vi "GUI_Scopes_v3.0.1.vi"() -> ()   [LabVIEW 2013]
uses:
  Device Drivers/PXIdigitizer/impedance_Enum_TypDEf.ctl
  Device Drivers/PXIdigitizer/coupling_Enum_TypDef.ctl
  Shared/type definition/trace_TypDef.ctl
  Device Drivers/shared/scopeTraceInfo_TypDEf.ctl
  Device Drivers/PXIdigitizer/mode_TypDef.ctl
  Device Drivers/PXIdigitizer/SignalFormat_TypDef.ctl
  Device Drivers/PXIdigitizer/triggerwindowmode2_TypDef.ctl
  Device Drivers/PXIdigitizer/TriggerSource_TypDef.ctl
  Shared/Device Driver/positive_negatice2_typDef.ctl
  Device Drivers/PXIdigitizer/coupling_TypDef.ctl
  Device Drivers/PXIdigitizer/TVEvent_TypDef.ctl
  Device Drivers/PXIdigitizer/Polarity_TypDEf.ctl
  Shared/Device Driver/OnOffTypeDef.ctl
  Device Drivers/PXIdigitizer/subVis/Trigger.DigitalSource_TypDEf.ctl
  Device Drivers/ScopeAnalysis/SubVis/method_TypDef.ctl
  Device Drivers/PXIdigitizer/subVis/channels_TypDef.ctl
  commandForScopeTrace.ctl
  <vilib>/Analysis/1siggen.llb/Ramp Pattern by Delta.vi
  <vilib>/Analysis/NI_AALBase.lvlib
panel:
  out "channelNames":refnum<vi>[](array[refnum])
  out "Number of channels":i32=8
  out "basic sub.":string="wait>>coupling.Channel1,coupling.Channel0,coupling.Channel2,coupling.Channel3,coupling.Channel4,coupling.Channel5,coupling.Channel6,coupling.Channel7,offset.Channel1,offset.Channel0,offset.Channel2,offset.Channel3,offset.Channel4,offset.Channel5,offset.Channel6,offset.Channel7,verticalrange.Channel1,verticalrange.Channel0,verticalrange.Channel2,verticalrange.Channel3,verticalrange.Channel4,verticalrange.Channel5,verticalrange.Channel6,verticalrange.Channel7,channelenabled.Channel1,channelenabled.Channel0,channelenabled.Channel2,channelenabled.Channel3,channelenabled.Channel4,channelenabled.Channel5,channelenabled.Channel6,channelenabled.Channel7,probeattenuation.Channel1,probeattenuation.Channel0,probeattenuation.Channel2,probeattenuation.Channel3,probeattenuation.Channel4,probeattenuation.Channel5,probeattenuation.Channel6,probeattenuation.Channel7,impedance.Channel1,impedance.Channel0,impedance.Channel2,impedance.Channel3,impedance.Channel4,impedance.Channel5,impedance.Channel6,impedance.Channel7,Names.Channel0,Names.Channel1,Names.Channel2,Names.Channel3,Names.Channel4,Names.Channel5,Names.Channel6,Names.Channel7,channelenabled.Channel0,channelenabled.Channel1,channelenabled.Channel2,channelenabled.Channel3,channelenabled.Channel4,channelenabled.Channel5,channelenabled.Channel6,channelenabled.Channel7,save,Horizontal.Enforce Realtime,Horizontal.Actual Record Length,Horizontal.Min Record Length,Horizontal.Actual Sample Rate,Horizontal.Min Sample Rate,Trigger.DC Restore,Trigger.Window Mode,Trigger.Polarity,Trigger.TV Event,Trigger.Coupling,Trigger.Slope,Trigger.AnalogSource,Trigger.High Level,Trigger.Low Level,Trigger.Hysteresis,Trigger.Delay,Trigger.Holdoff,Trigger.Signal Format,Trigger.Line Number,Trigger.Mode,Trigger.DigitalSource,"
  out "Channel NAmes":string[](array[string])
  out "show3 array":refnum<vi>[](array[refnum])
  out "showAll array":refnum<vi>[](array[refnum])
  out "enabled array":refnum<vi>[](array[refnum])
  out "wavegaph array":refnum<vi>[](array[refnum])
  out "traces array":refnum<vi>[](array[refnum])
  in  "save":T1
  out "horizontal ref":refnum<vi>[](array[refnum])
  out "Trigger ref":refnum<vi>[](array[refnum])
  out "indecator ref array":refnum<vi>[](array[refnum])
  in  "time to wait (TCP) 2":i32=10
  in  "plot":bool=TRUE
  out "ratio(h)":bool
  out "fixsize":bool
  in  "shotnumber":i32
  out "error (h)":bool
  in  "scopeTraceGUI.Channel7":T2
  in  "scopeTraceGUI.Channel6":T2
  in  "scopeTraceGUI.Channel4":T2
  in  "scopeTraceGUI.Channel3":T2
  in  "scopeTraceGUI.Channel5":T2
  in  "scopeTraceGUI.Channel2":T2
  out "Device Name (h)":string="TS-digitizer-1"
  in  "Main Tap":T4(tab)
  out "channel 1":waveform(dbl)(graph)
  in  "Tab Control":T5(tab)
  in  "coupling":T6=enum."DC"
  in  "channelenabled":enum16{"off", "on"}(ring)=enum."on"
  in  "offset":dbl
  in  "verticalrange":dbl=6.0
  in  "probeattenuation":dbl=1.0
  in  "impedance":T7=enum."50 ohms"
  in  "Channel":T8(ring)
  in  "ChannelRing":u16(ring) items=["Ch1", "Ch2", "Ch3", "Ch4", "Ch5", "Ch6", "Ch7", "Ch8"]
  in  "Horizontal.Min Sample Rate":dbl=6000000.0 step=1000000.0 format="%.2p"
  in  "Horizontal.Min Record Length":i32=10000 format="%.0p"
  out "Horizontal.Actual Record Length":i32=10000
  out "Horizontal.Actual Sample Rate":dbl=6000000.0 format="%.2p"
  in  "Horizontal.Enforce Realtime":T1=enum."on"
  out "time wimdow":dbl=0.0016666666666666668 format="%#_6p"
  out "resolution":dbl=1.6666666666666668e-07 format="%#_6p"
  in  "Trigger.Delay":dbl min=-0.001 max=0.001 step=1e-08 format="%#_12e"
  in  "Trigger.Coupling":T9=enum."DC" caption="Coupling"
  in  "Trigger.Mode":T10=enum."Digital Edge"
  in  "Trigger.Polarity":T11=enum."Positive" caption="Polarity"
  in  "Trigger.Line Number":i32=1
  in  "Trigger.Signal Format":T12 caption="Signal Format"
  in  "Trigger.DC Restore":T1
  in  "Trigger.TV Event":T13=enum."Any Line" caption="TV Event"
  in  "Trigger.Holdoff":dbl
  in  "Trigger.AnalogSource":T14
  in  "Trigger.Low Level":dbl=0.5
  in  "Trigger.Slope":T15 caption="Slope"
  in  "Trigger.High Level":dbl=1.0
  in  "Trigger.Hysteresis":dbl=0.05
  in  "Trigger.Window Mode":T16 caption="Window Mode"
  in  "Trigger.DigitalSource":T17=enum."PFI 1"
  out "Names.Channel2":string="Ch3"
  out "Names.Channel3":string="Ch4"
  out "Names.Channel4":string="Ch5"
  out "Names.Channel5":string="Ch6"
  out "Names.Channel6":string="Ch7"
  out "Names.Channel7":string="Ch8"
  in  "show.2":T8(ring)=enum."Channel1"
  in  "show.Channel0":bool=TRUE
  in  "show.Channel1":bool=TRUE
  in  "show.Channel2":bool
  in  "show.Channel3":bool
  in  "show.Channel4":bool
  in  "show.Channel5":bool
  in  "show.Channel6":bool
  in  "show.Channel7":bool
  in  "channelenabled.Channel0":bool=TRUE
  in  "Y scale from range":bool
  in  "channelenabled.Channel1":bool=TRUE
  in  "channelenabled.Channel2":bool=TRUE
  in  "channelenabled.Channel3":bool=TRUE
  in  "channelenabled.Channel4":bool=TRUE
  in  "channelenabled.Channel5":bool=TRUE
  in  "channelenabled.Channel6":bool=TRUE
  in  "channelenabled.Channel7":bool=TRUE
  in  "show.1":T8(ring)
  in  "Display":enum32{"All", "3Channels"}(radio)
  out "Names.Channel0":string="Ch1"
  out "Names.Channel1":string="Ch2"
  in  "Calculations.Additional.Analysis2":dbl=0.5
  in  "Calculations.Additional.Analysis1":dbl=0.5
  in  "Calculations.Method.Analysis2":T18 caption="Method"
  in  "Calculations.Linked.Analysis2":T19
  out "Measurements.Analysis2":dbl=0.5
  in  "Calculations.Method.Analysis1":T18 caption="Method"
  in  "Calculations.Linked.Analysis1":T19
  out "Measurements.Analysis1":dbl=0.5
  in  "scopeTraceGUI.Channel0":T2
  in  "scopeTraceGUI.Channel1":T2
  out "channel 0":waveform(dbl)(graph)
  out "All Channel":waveform(dbl)[](graph)
  out "local Port":u16=65442
  out "port or service name":u16=65445
  out "Remote Host":string="192.168.10.21"
  in  "timeout ms (slow resp)":i32=500
  in  "reset":bool
  out "image con closed":bool
  out "image \nconnection":bool
  out "image con closed 2":bool
  out "All Devices (h)":string[](array[string])=["PIXIFake", "TREX PXI fast", "TREX PXI slow", "TS-digitizer-1"]
  in  "time to wait (TCP)":i32=10
  out "error out":errorcluster
  out "connections (hidden)":variant[](array[variant])=[variant(refnum<k16> refnum), variant(refnum<k16> refnum)]
  in  "time to wait (main loop)":i32=200
  out "Data String":string="coupling.Channel1,DC\r\ncoupling.Channel0,DC\r\ncoupling.Channel2,DC\r\ncoupling.Channel3,DC\r\ncoupling.Channel4,DC\r\ncoupling.Channel5,DC\r\ncoupling.Channel6,DC\r\ncoupling.Channel7,DC\r\noffset.Channel1,0.000000000000\r\noffset.Channel0,0.000000000000\r\noffset.Channel2,0.000000000000\r\noffset.Channel3,0.000000000000\r\noffset.Channel4,0.000000000000\r\noffset.Channel5,0.000000000000\r\noffset.Channel6,0.000000000000\r\noffset.Channel7,0.000000000000\r\nverticalrange.Channel1,6.000000000000\r\nverticalrange.Channel0,6.000000000000\r\nverticalrange.Channel2,6.000000000000\r\nverticalrange.Channel3,6.000000000000\r\nverticalrange.Channel4,6.000000000000\r\nverticalrange.Channel5,6.000000000000\r\nverticalrange.Channel6,6.000000000000\r\nverticalrange.Channel7,6.000000000000\r\nchannelenabled.Channel1,on\r\nchannelenabled.Channel0,on\r\nchannelenabled.Channel2,on\r\nchannelenabled.Channel3,on\r\nchannelenabled.Channel4,on\r\nchannelenabled.Channel5,on\r\nchannelenabled.Channel6,on\r\nchannelenabled.Channel7,on\r\nprobeattenuation.Channel1,1.000000000000\r\nprobeattenuation.Channel0,1.000000000000\r\nprobeattenuation.Channel2,1.000000000000\r\nprobeattenuation.Channel3,1.000000000000\r\nprobeattenuation.Channel4,1.000000000000\r\nprobeattenuation.Channel5,1.000000000000\r\nprobeattenuation.Channel6,1.000000000000\r\nprobeattenuation.Channel7,1.000000000000\r\nimpedance.Channel1,50 ohms\r\nimpedance.Channel0,50 ohms\r\nimpedance.Channel2,50 ohms\r\nimpedance.Channel3,50 ohms\r\nimpedance.Channel4,50 ohms\r\nimpedance.Channel5,50 ohms\r\nimpedance.Channel6,50 ohms\r\nimpedance.Channel7,50 ohms\r\nNames.Channel0,Ch1\r\nNames.Channel1,Ch2\r\nNames.Channel2,Ch3\r\nNames.Channel3,Ch4\r\nNames.Channel4,Ch5\r\nNames.Channel5,Ch6\r\nNames.Channel6,Ch7\r\nNames.Channel7,Ch8\r\nchannelenabled.Channel0,on\r\nchannelenabled.Channel1,on\r\nchannelenabled.Channel2,on\r\nchannelenabled.Channel3,on\r\nchannelenabled.Channel4,on\r\nchannelenabled.Channel5,on\r\nchannelenabled.Channel6,on\r\nchannelenabled.Channel7,on\r\nsave,off\r\nHorizontal.Enforce Realtime,on\r\nHorizontal.Actual Record Length,10000.000000000000\r\nHorizontal.Min Record Length,10000.000000000000\r\nHorizontal.Actual Sample Rate,6000000.000000000000\r\nHorizontal.Min Sample Rate,6000000.000000000000\r\nTrigger.DC Restore,off\r\nTrigger.Window Mode,Entering\r\nTrigger.Polarity,Positive\r\nTrigger.TV Event,Any Line\r\nTrigger.Coupling,DC\r\nTrigger.Slope,Positive\r\nTrigger.AnalogSource,Channel 0\r\nTrigger.High Level,1.000000000000\r\nTrigger.Low Level,0.500000000000\r\nTrigger.Hysteresis,0.050000000000\r\nTrigger.Delay,0.000000000000\r\nTrigger.Holdoff,0.000000000000\r\nTrigger.Signal Format,M-NTSC\r\nTrigger.Line Number,1.000000000000\r\nTrigger.Mode,Digital Edge\r\nTrigger.DigitalSource,PFI 1\r\n"
  in  "Local Saving Path":path
  out "concatenated string":string="wait>>coupling.Channel1,coupling.Channel0,coupling.Channel2,coupling.Channel3,coupling.Channel4,coupling.Channel5,coupling.Channel6,coupling.Channel7,offset.Channel1,offset.Channel0,offset.Channel2,offset.Channel3,offset.Channel4,offset.Channel5,offset.Channel6,offset.Channel7,verticalrange.Channel1,verticalrange.Channel0,verticalrange.Channel2,verticalrange.Channel3,verticalrange.Channel4,verticalrange.Channel5,verticalrange.Channel6,verticalrange.Channel7,channelenabled.Channel1,channelenabled.Channel0,channelenabled.Channel2,channelenabled.Channel3,channelenabled.Channel4,channelenabled.Channel5,channelenabled.Channel6,channelenabled.Channel7,probeattenuation.Channel1,probeattenuation.Channel0,probeattenuation.Channel2,probeattenuation.Channel3,probeattenuation.Channel4,probeattenuation.Channel5,probeattenuation.Channel6,probeattenuation.Channel7,impedance.Channel1,impedance.Channel0,impedance.Channel2,impedance.Channel3,impedance.Channel4,impedance.Channel5,impedance.Channel6,impedance.Channel7,Names.Channel0,Names.Channel1,Names.Channel2,Names.Channel3,Names.Channel4,Names.Channel5,Names.Channel6,Names.Channel7,channelenabled.Channel0,channelenabled.Channel1,channelenabled.Channel2,channelenabled.Channel3,channelenabled.Channel4,channelenabled.Channel5,channelenabled.Channel6,channelenabled.Channel7,save,Horizontal.Enforce Realtime,Horizontal.Actual Record Length,Horizontal.Min Record Length,Horizontal.Actual Sample Rate,Horizontal.Min Sample Rate,Trigger.DC Restore,Trigger.Window Mode,Trigger.Polarity,Trigger.TV Event,Trigger.Coupling,Trigger.Slope,Trigger.AnalogSource,Trigger.High Level,Trigger.Low Level,Trigger.Hysteresis,Trigger.Delay,Trigger.Holdoff,Trigger.Signal Format,Trigger.Line Number,Trigger.Mode,Trigger.DigitalSource,"
  out "error message":string
  out "Data Connection out":bool=TRUE
  # "enabled"
  # "show"
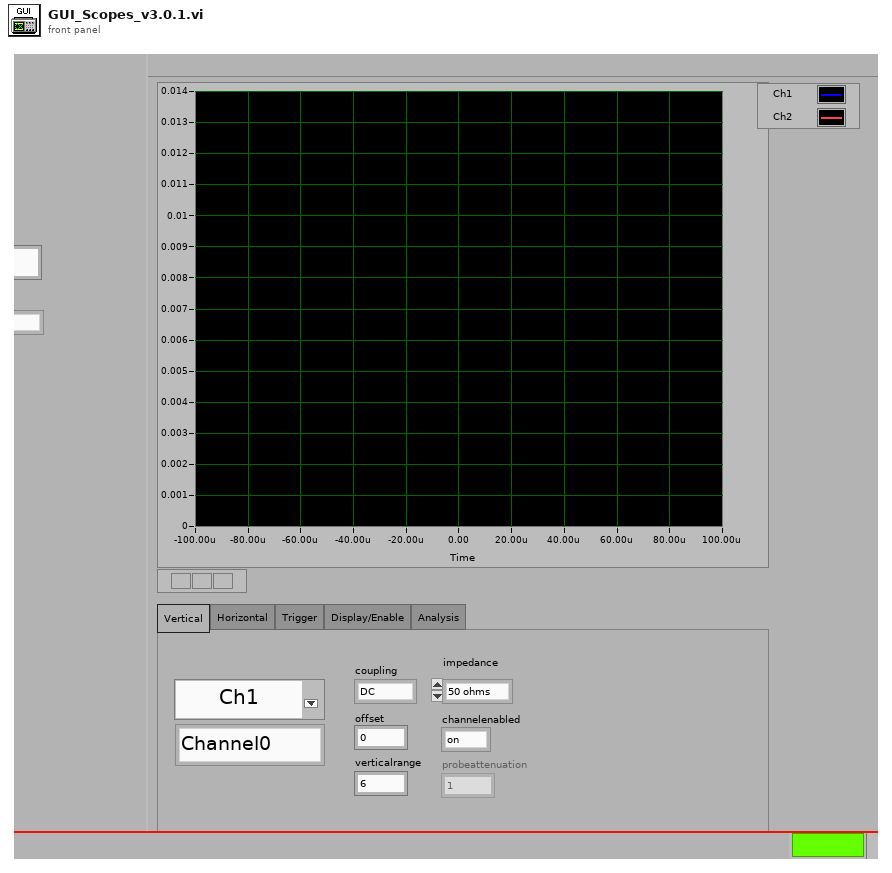
[diagram p1: front panel]
types:
  T1 = typedef "OnOffTypeDef.ctl" = enum16{"off", "on"}
  T2 = typedef "trace_TypDef.ctl" = cluster{"info":T3, "wfm":dbl[]}
  T3 = typedef "scopeTraceInfo_TypDEf.ctl" = cluster{"Name":string, "N":dbl, "t0":dbl, "dt":dbl, "offset":dbl, "gain":dbl, "coupling":string, "impedance":string, "range":dbl}
  T4 = enum32{"All Channels", "Network", "Internal", "Advanced"}
  T5 = enum32{"Vertical", "Horizontal", "Trigger", "Display/Enable", "Analysis"}
  T6 = typedef "coupling_Enum_TypDef.ctl" = enum16{"AC", "DC", "Ground"}
  T7 = typedef "impedance_Enum_TypDEf.ctl" = enum16{"1 mega ohm", "<NA>", "50 ohms"}
  T8 = enum16{"Channel0", "Channel1", "Channel2", "Channel3", "Channel4", "Channel5", "Channel6", "Channel7"}
  T9 = typedef "coupling_TypDef.ctl" = enum16{"AC", "DC", "HF Reject", "LF Reject", "AC Plus HF Reject"}
  T10 = typedef "mode_TypDef.ctl" = enum32{"Immediate", "Analog Edge", "Analog Window", "Analog Hysteresis", "Video", "Digital Edge"}
  T11 = typedef "Polarity_TypDEf.ctl" = enum16{"Negative", "Positive"}
  T12 = typedef "SignalFormat_TypDef.ctl" = enum16{"M-NTSC", "B/G-PAL", "SECAM", "M-PAL", "480i/59.94 fps", "480i/60 fps", "480p/59.94 Fps", "480p/60 Fps", "576i/50 fps", "576p/50 Fps", "720p/50 Fps", "720p/59.94 Fps", "720p/60 Fps", "1080i/50 fps", "1080i/59.94 fps", "1080i/60 fps", "1080p/24 Fps"}
  T13 = typedef "TVEvent_TypDef.ctl" = enum16{"Field 1", "Field 2", "Any Field", "Any Line", "Line Number"}
  T14 = typedef "TriggerSource_TypDef.ctl" = enum16{"Channel 0", "Channel 1", "Channel 2", "Channel 3", "Channel 4", "Channel 5", "Channel 6", "Channel 7", "External TRIG"}
  T15 = typedef "positive_negatice2_typDef.ctl" = enum16{"Positive", "Negative"}
  T16 = typedef "triggerwindowmode2_TypDef.ctl" = enum16{"Entering", "Leaving"}
  T17 = typedef "Trigger.DigitalSource_TypDEf.ctl" = enum16{"RTSI 0", "RTSI 1", "RTSI 2", "RTSI 3", "RTSI 4", "RTSI 5", "RTSI 6", "PFI 0", "PFI 1", "PFI 2", "PXI Star Trigger"}
  T18 = typedef "method_TypDef.ctl" = enum16{"n/a", "max", "min", "energy", "trigger", "maxtime", "mintime"}
  T19 = typedef "channels_TypDef.ctl" = enum16{"Channel0", "Channel1", "Channel2", "Channel3", "Channel4", "Channel5", "Channel6", "Channel7", "n/a"}
  T20 = typedef "commandForScopeTrace.ctl" = enum16{"get", "set", "init", "get ALL"}
  T21 = typedef "scopeTrace_TypDef.ctl" = cluster{"Info":cluster{"t0":dbl, "dt":dbl, "gain":dbl, "Name":string, "offset":dbl}, "Data":i16[]}
  T22 = cluster{"t0":dbl, "dt":dbl, "gain":dbl, "Name":string, "offset":dbl}
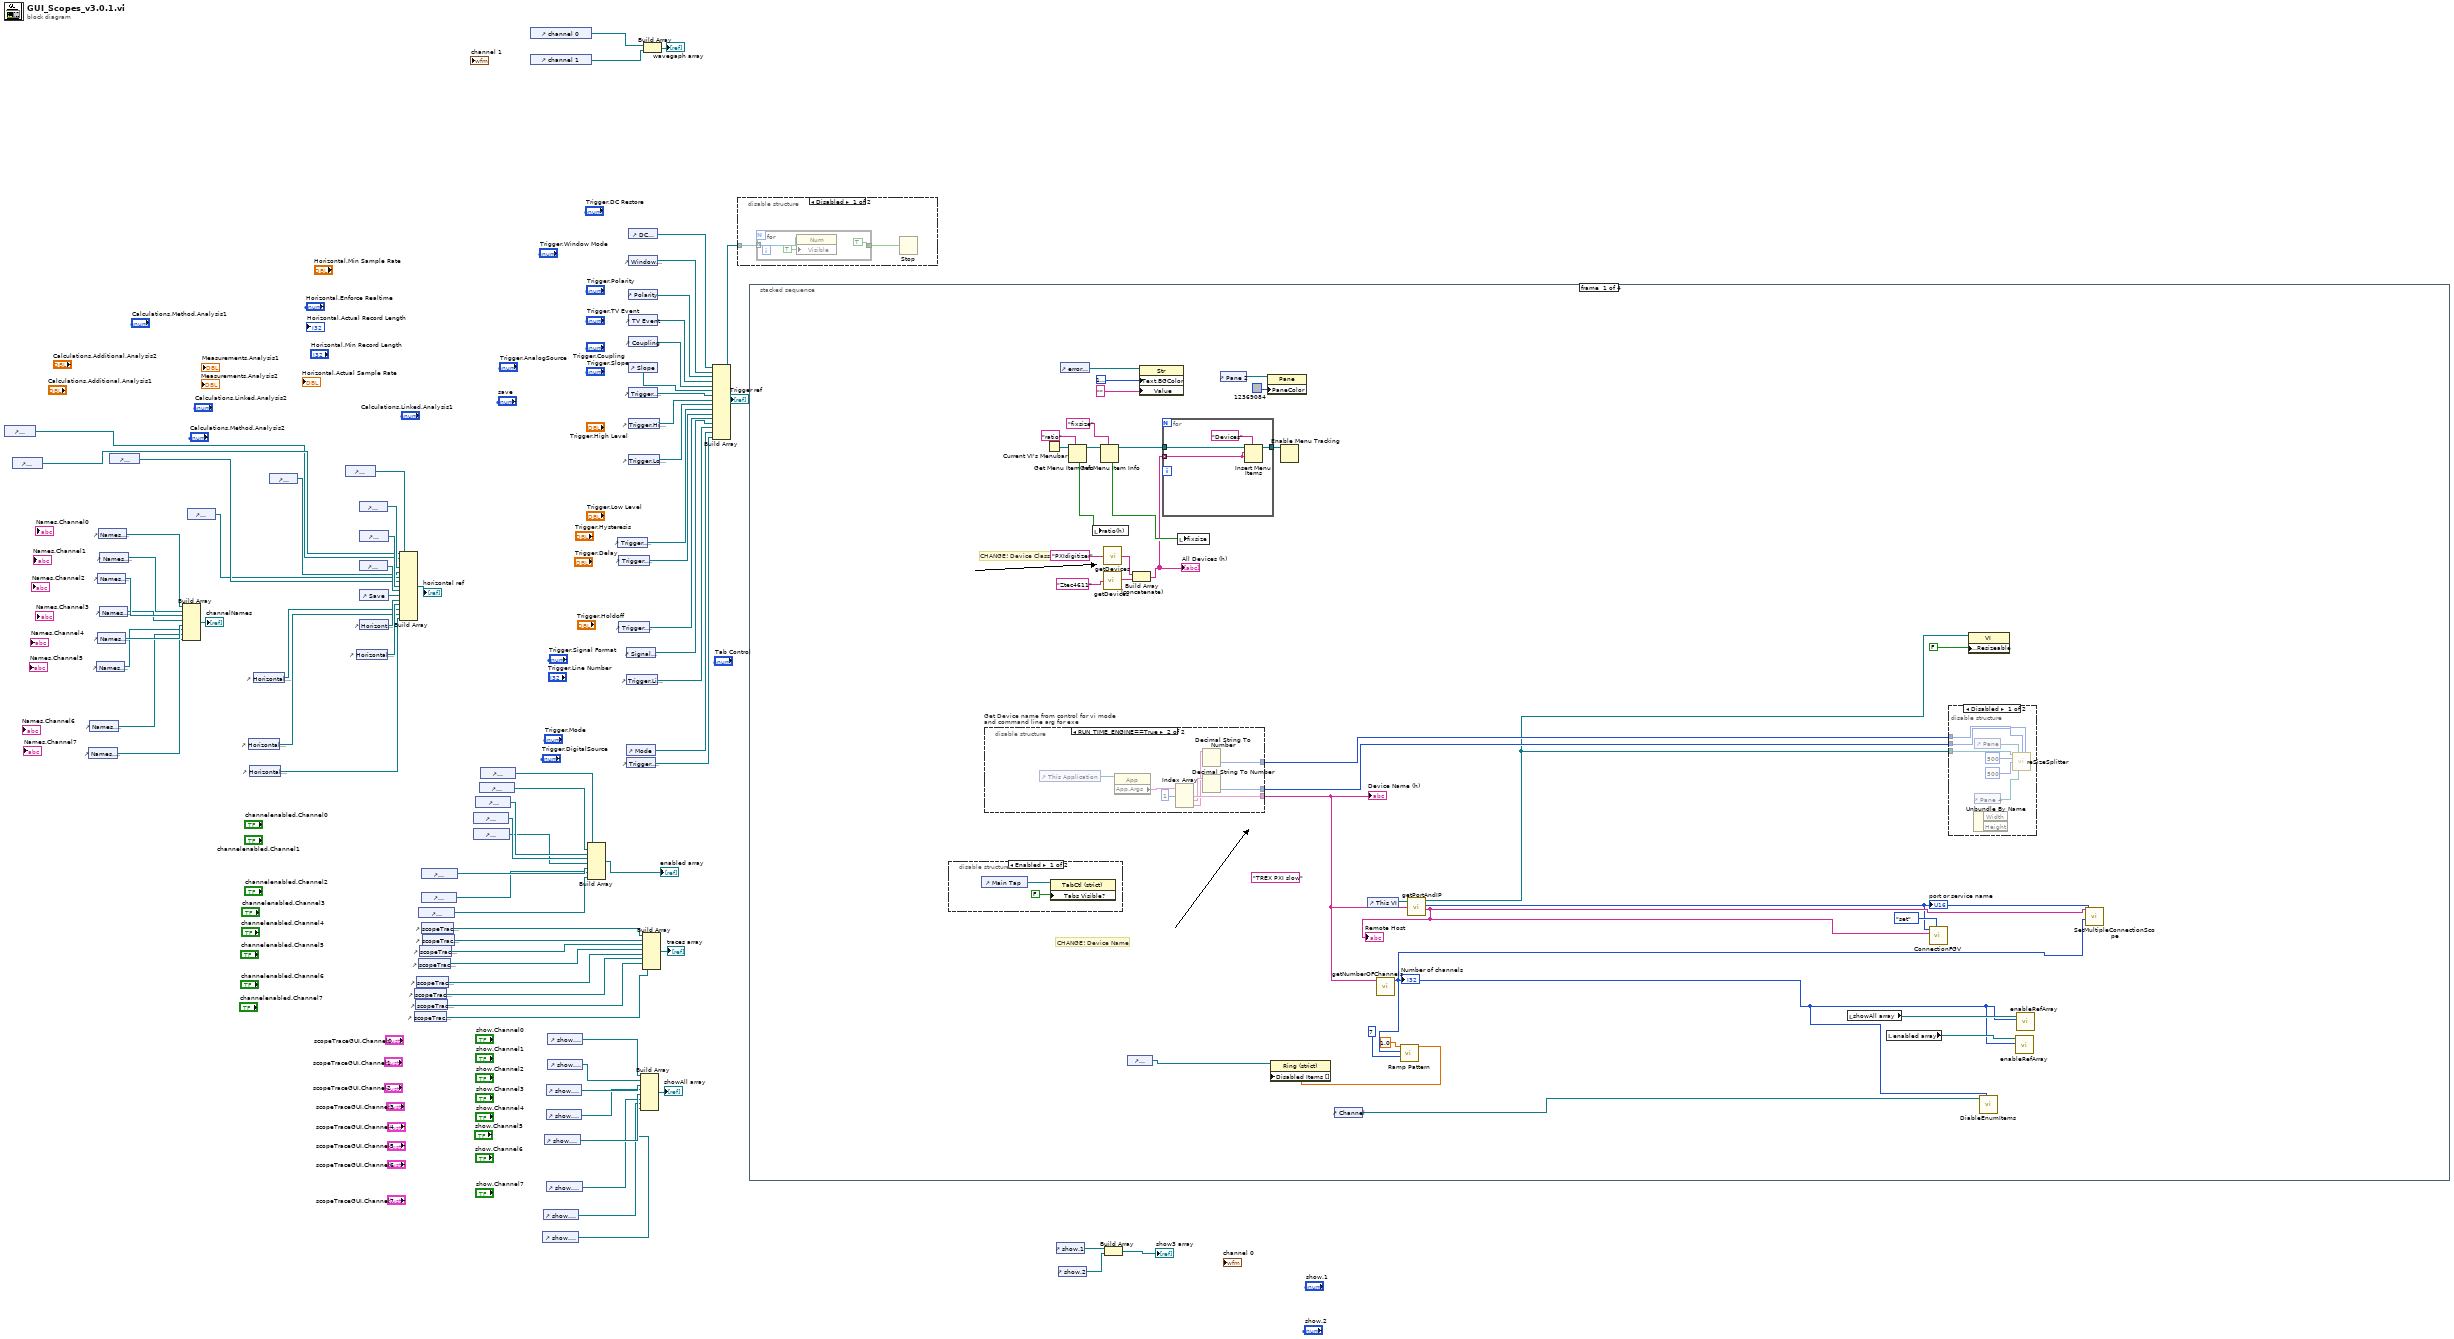
[diagram p0: block diagram]
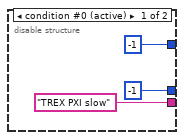
[diagram p5: hidden frame]
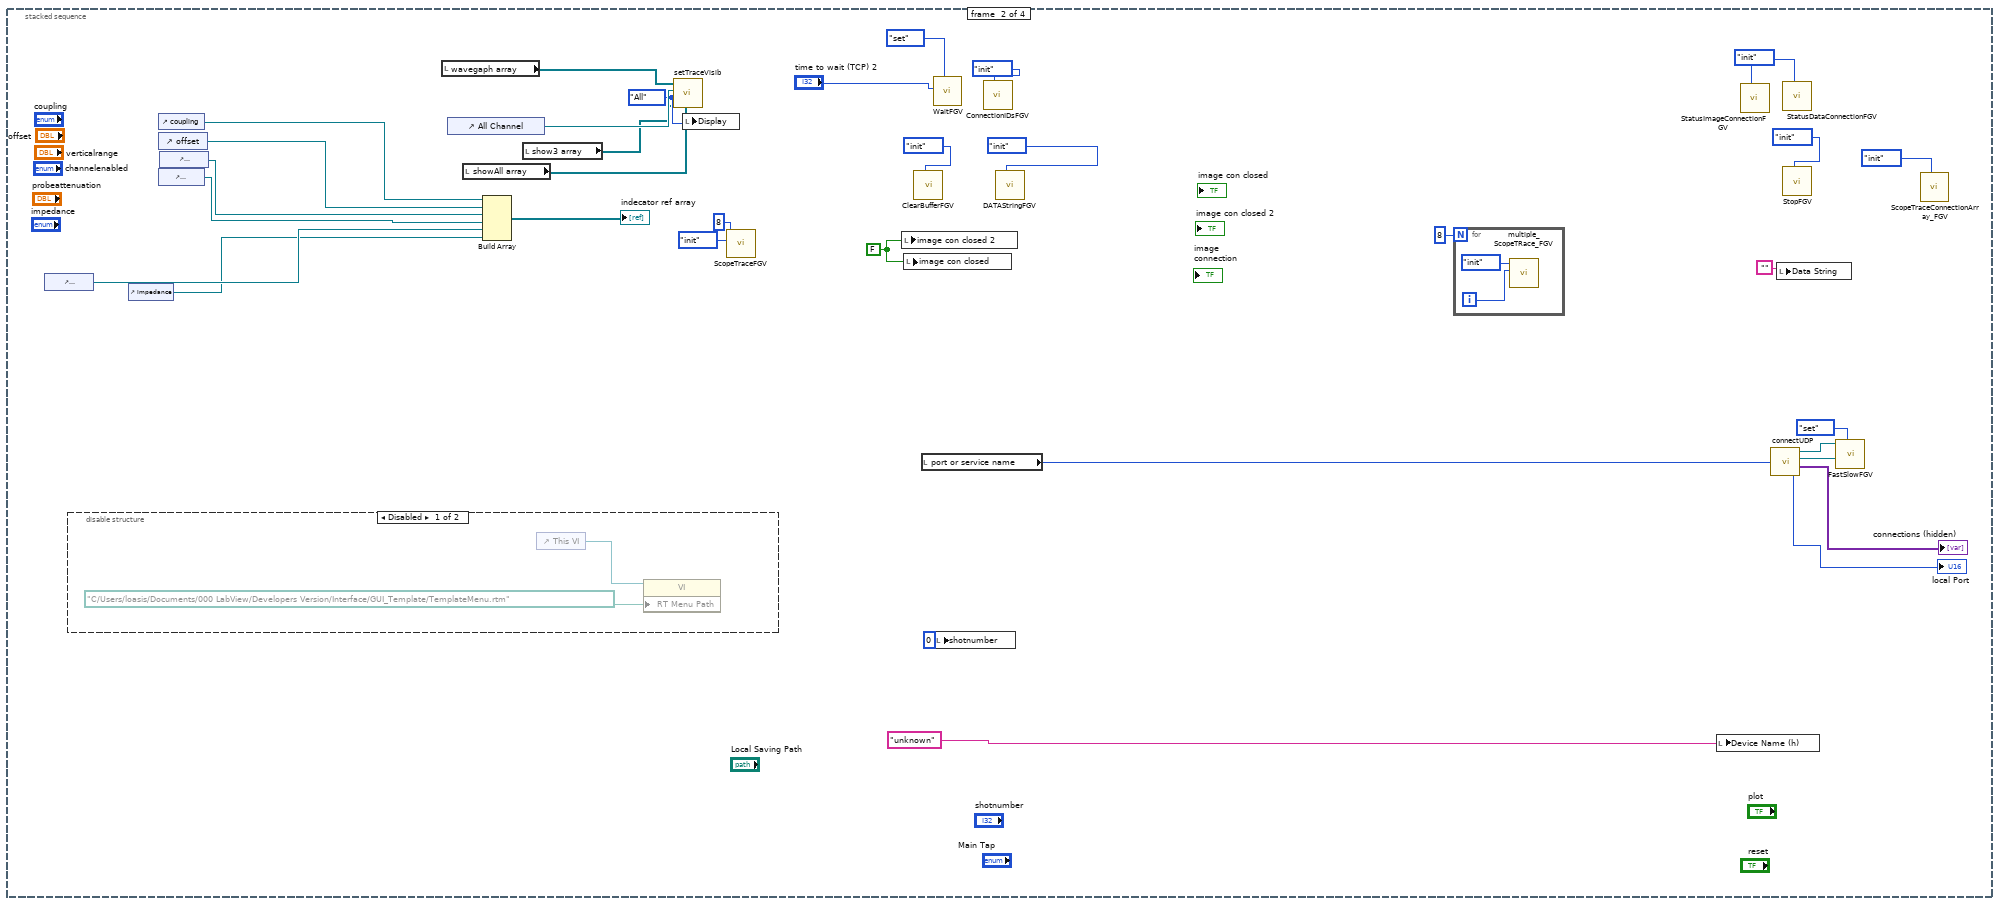
[diagram p6: hidden frame]
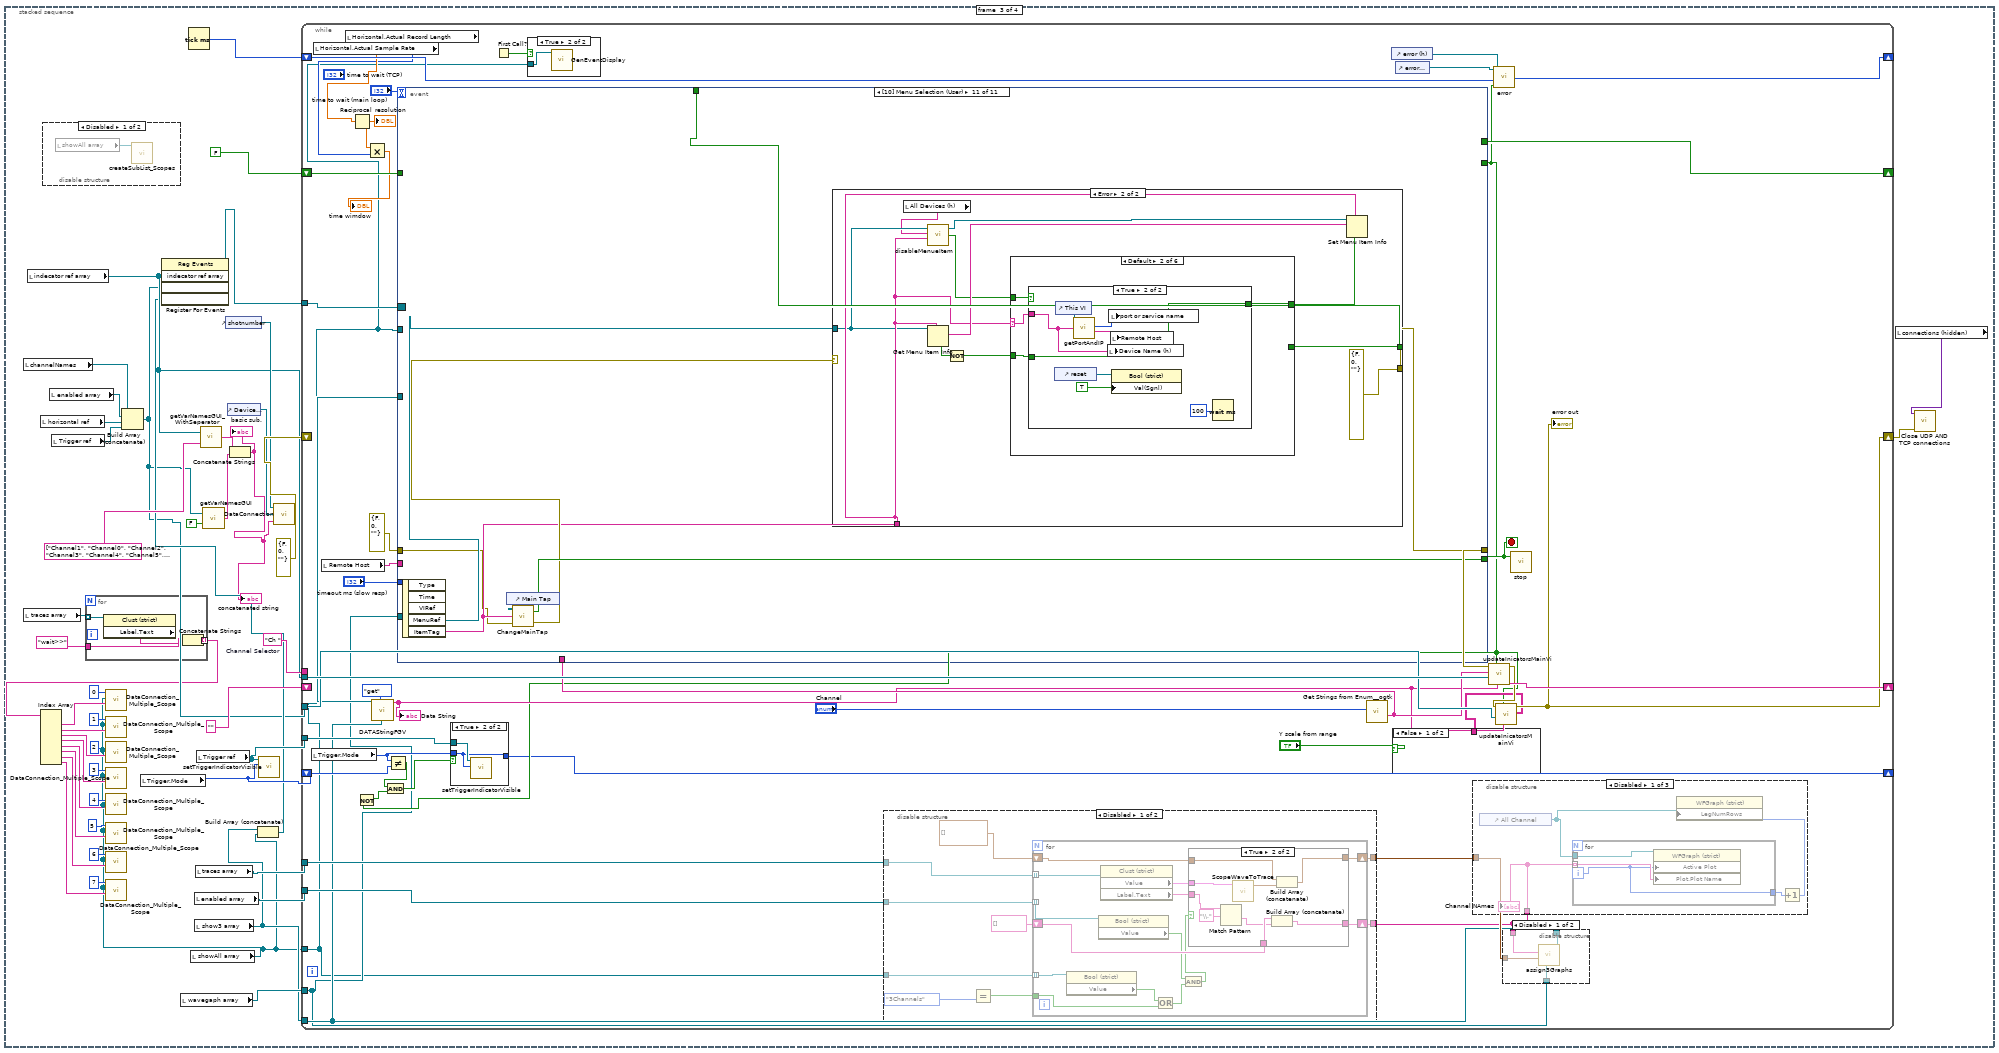
[diagram p8: hidden frame]
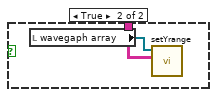
[diagram p17: hidden frame]
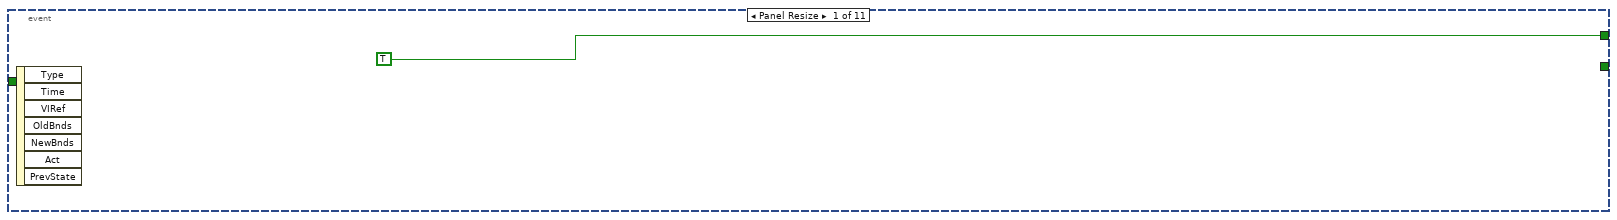
[diagram p18: hidden frame]
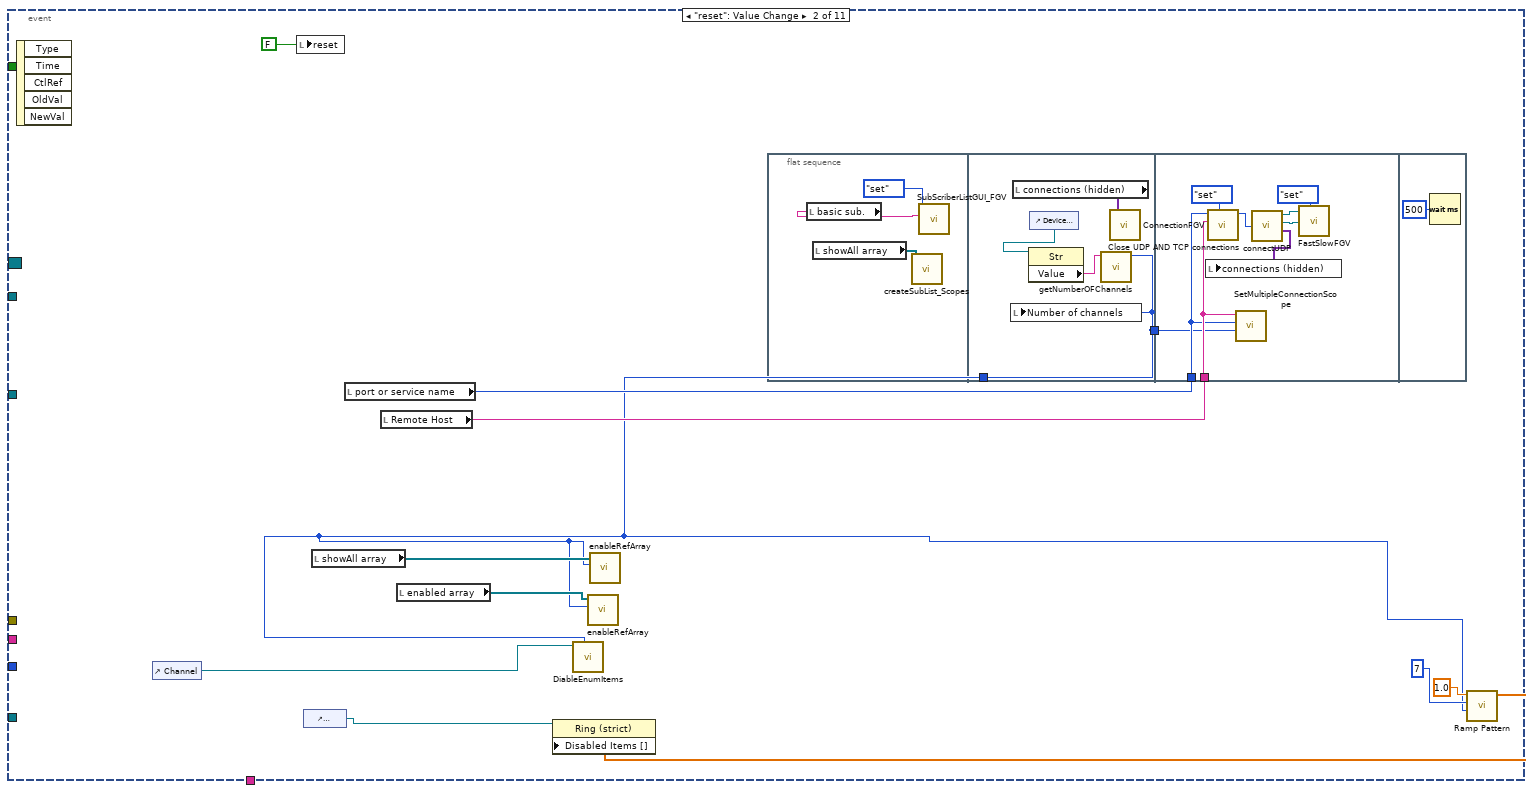
[diagram p19: hidden frame]
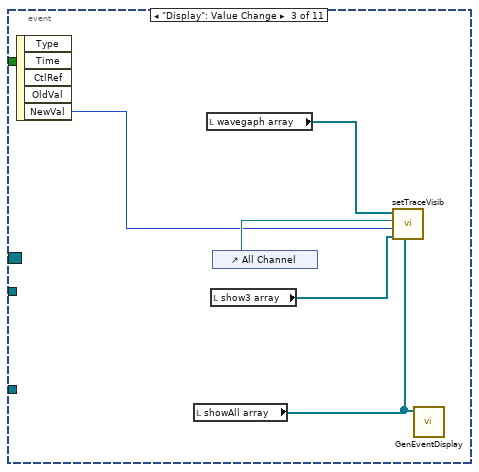
[diagram p20: hidden frame]
diagram:
  n1 = control-ref of="Calculations.Additional.Analysis1"() -> (w1:refnum<vi>)
  n2 = control-ref of="Calculations.Additional.Analysis2"() -> (w2:refnum<vi>)
  n3 = control-ref of="Names.Channel7"() -> (w11:refnum<vi>)
  n4 = control-ref of="Names.Channel6"() -> (w12:refnum<vi>)
  n5 = control-ref of="Names.Channel5"() -> (w13:refnum<vi>)
  n6 = control-ref of="Names.Channel2"() -> (w16:refnum<vi>)
  n7 = control-ref of="Names.Channel4"() -> (w14:refnum<vi>)
  n8 = control-ref of="Names.Channel0"() -> (w18:refnum<vi>)
  n9 = control-ref of="Names.Channel3"() -> (w15:refnum<vi>)
  n10 = control-ref of="Names.Channel1"() -> (w17:refnum<vi>)
  n11 = control-ref of="Measurements.Analysis1"() -> (w7:refnum<vi>)
  n12 = Build Array(w18, w17, w16, w15, w14, w13, w12, w11) -> (→"channelNames":refnum<vi>[])
  n13 = control-ref of="LinkedChannel.M2"() -> (w4:refnum<vi>)
  n14 = control-ref of="Horizontal.Actual Sample Rate"() -> (w56:refnum<vi>)
  n15 = control-ref of="Horizontal.Min Sample Rate"() -> (w54:refnum<vi>)
  n16 = control-ref of="Horizontal.Min Record Length"() -> (w57:refnum<vi>)
  n17 = control-ref of="LinkedChannel.M2"() -> (w5:refnum<vi>)
  n18 = control-ref of="Measurements.Analysis2"() -> (w3:refnum<vi>)
  n19 = control-ref of="Horizontal.Actual Record Length"() -> (w58:refnum<vi>)
  n20 = control-ref of="Calculations.Method.Analysis2"() -> (w6:refnum<vi>)
  n21 = control-ref of="Calculations.Method.Analysis1"() -> (w9:refnum<vi>)
  n22 = control-ref of="LinkedChannel.M1"() -> (w8:refnum<vi>)
  n23 = control-ref of="Save"() -> (w52:refnum<vi>)
  n24 = control-ref of="Horizontal.Enforce Realtime"() -> (w59:refnum<vi>)
  n25 = Build Array(w2, w1, w3, w6, w5, w4, w7, w8, w9, w52, w59, w58, w57, w56, w54) -> (→"horizontal ref":refnum<vi>[])
  n26 = control-ref of="scopeTrace.Channel7"() -> (w43:refnum<vi>)
  n27 = control-ref of="scopeTrace.Channel5"() -> (w45:refnum<vi>)
  n28 = control-ref of="scopeTrace.Channel6"() -> (w44:refnum<vi>)
  n29 = control-ref of="scopeTrace.Channel4"() -> (w46:refnum<vi>)
  n30 = control-ref of="scopeTrace.Channel3"() -> (w47:refnum<vi>)
  n31 = control-ref of="channelenabled.Channel7"() -> (w34:refnum<vi>)
  n32 = control-ref of="scopeTrace.Channel2"() -> (w48:refnum<vi>)
  n33 = control-ref of="channelenabled.Channel6"() -> (w35:refnum<vi>)
  n34 = control-ref of="channelenabled.Channel5"() -> (w36:refnum<vi>)
  n35 = control-ref of="scopeTrace.Channel0"() -> (w33:refnum<vi>)
  n36 = control-ref of="scopeTrace.Channel1"() -> (w32:refnum<vi>)
  n37 = control-ref of="channelenabled.Channel3"() -> (w38:refnum<vi>)
  n38 = control-ref of="channelenabled.Channel4"() -> (w37:refnum<vi>)
  n39 = control-ref of="channelenabled.Channel2"() -> (w39:refnum<vi>)
  n40 = control-ref of="channelenabled.Channel1"() -> (w40:refnum<vi>)
  n41 = control-ref of="channelenabled.Channel0"() -> (w42:refnum<vi>)
  n42 = control-ref of="channel 1"() -> (w19:refnum<vi>)
  n43 = control-ref of="channel 0"() -> (w50:refnum<vi>)
  n44 = control-ref of="show.Channel7"() -> (w24:refnum<vi>)
  n45 = control-ref of="show.Channel6"() -> (w25:refnum<vi>)
  n46 = control-ref of="show.Channel4"() -> (w27:refnum<vi>)
  n47 = control-ref of="show.Channel2"() -> (w29:refnum<vi>)
  n48 = control-ref of="show.Channel3"() -> (w28:refnum<vi>)
  n49 = control-ref of="show.Channel5"() -> (w26:refnum<vi>)
  n50 = control-ref of="show.Channel0"() -> (w31:refnum<vi>)
  n51 = control-ref of="show.Channel1"() -> (w30:refnum<vi>)
  n52 = Build Array(w42, w40, w39, w38, w37, w36, w35, w34) -> (→"enabled array":refnum<vi>[])
  n53 = control-ref of="Trigger.Hysteresis"() -> (w66:refnum<vi>)
  n54 = control-ref of="Trigger.Holdoff"() -> (w64:refnum<vi>)
  n55 = control-ref of="Trigger.Delay"() -> (w65:refnum<vi>)
  n56 = control-ref of="Signal Format"() -> (w63:refnum<vi>)
  n57 = control-ref of="Trigger.Line Number"() -> (w62:refnum<vi>)
  n58 = control-ref of="Mode"() -> (w61:refnum<vi>)
  n59 = control-ref of="Trigger.DigitalSource"() -> (w60:refnum<vi>)
  n60 = control-ref of="DC Restore"() -> (w75:refnum<vi>)
  n61 = control-ref of="Window Mode"() -> (w74:refnum<vi>)
  n62 = control-ref of="Polarity"() -> (w73:refnum<vi>)
  n63 = control-ref of="TV Event"() -> (w72:refnum<vi>)
  n64 = control-ref of="Coupling"() -> (w71:refnum<vi>)
  n65 = control-ref of="Slope"() -> (w70:refnum<vi>)
  n66 = control-ref of="Trigger.AnalogSource"() -> (w69:refnum<vi>)
  n67 = control-ref of="Trigger.High Level"() -> (w68:refnum<vi>)
  n68 = control-ref of="Trigger.Low Level"() -> (w67:refnum<vi>)
  n69 = Build Array(w31, w30, w29, w28, w27, w26, w25, w24) -> (→"showAll array":refnum<vi>[])
  n70 = Build Array(w33, w32, w48, w47, w46, w45, w44, w43) -> (→"traces array":refnum<vi>[])
  n71 = Build Array(w50, w19) -> (→"wavegaph array":refnum<vi>[])
  n72 = Build Array(w75, w74, w73, w72, w71, w70, w69, w68, w67, w66, w65, w64, w63, w62, w61, w60) -> (w53:refnum<vi>[])
  "Trigger ref" <- w53
  n73 = disable-structure shown="Disabled" {
    disable-tunnel: w53 -> [w77 _]
    frame Disabled {
      n74 = for {
        tunnel: w77 -> [w80] mode=indexing
        tunnel: [TRUE] -> w76
        n75 = property class="Num"(reference=w80, "Visible"=TRUE) -> ()  [unwired: 1 in, 2 out]
      }
      n76 = Stop(stop? (T)=w76) -> ()
    }
    frame Enabled {
    }
  }
  n77 = stacked-sequence {
    frame #0 {
      (unwired) "TREX PXI slow" ("Device Name for vi mode")
      # "CHANGE! Device Name"
      # "CHANGE! Device Class"
      n78 = disable-structure shown="Enabled" {
        frame Enabled {
          n79 = control-ref of="Main Tap"() -> (w117:refnum<vi>)
          n80 = property class="TabCtl (strict)"(reference=w117, "Tabs Visible?"=FALSE) -> ()  [unwired: 1 in, 2 out]
        }
        frame Disabled {
        }
      }
      n81 = disable-structure "Get Device name from control for vi mode\nand command line arg for exe" shown="RUN_TIME_ENGINE==True" {
        disable-tunnel: ["TREX PXI slow" ("Device Name for vi mode") w136] -> w93
        disable-tunnel: [i16 -1 ("left") w133] -> w115
        disable-tunnel: [i16 -1 ("left") w132] -> w114
        frame condition #0 (active) {
        }
        frame condition #1 {
          n82 = control-ref of="This Application"() -> (w139:refnum<vi>)
          n83 = property class="App"(reference=w139) -> ("App.Args"=w138:string[])  [unwired: 1 in, 2 out]
          n84 = Index Array(array=w138, index #1=1 ("index")) -> (element #1=w136:string, element #2=w135:string, element #3=w134:string)  [unwired: 2 in]
          n85 = Decimal String To Number(string=w134) -> (number=w132:i32)  [unwired: 2 in, 1 out]
          n86 = Decimal String To Number(string=w135) -> (number=w133:i32)  [unwired: 2 in, 1 out]
        }
      }
      "Device Name (h)" <- w93
      n87 = Current VI's Menubar() -> (w108:refnum<k9>)
      n88 = control-ref of="error message"() -> (w102:refnum<vi>)
      n89 = Get Menu Item Info(7:"ratio" ("item tag"), 11:w108) -> (3:w106:refnum<k9>, 4:w107:bool)  [unwired: 1 in, 5 out]
      n90 = local write "ratio(h)"(w107) -> ()
      n91 = Get Menu Item Info(7:"fixsize" ("item tag"), 11:w106) -> (3:w98:refnum<k9>, 4:w104:bool)  [unwired: 1 in, 5 out]
      n92 = call "getDevices.vi"("Device Class"="Ztec4611") -> ("All Devices"=w82:string[])
      n93 = call "getDevices.vi"("Device Class"="PXIdigitizer") -> ("All Devices"=w83:string[])
      n94 = control-ref of="ChannelRing"() -> (w89:refnum<vi>)
      n95 = Build Array (concatenate)(w83, w82) -> (w81:string[])
      "All Devices (h)" <- w81
      n96 = property class="Str"(reference=w102, "Text.BGColor"=u32 16777238, "Value"="") -> ()  [unwired: 1 in, 2 out]
      n97 = for {
        tunnel: w98 -> [w121]
        tunnel: [w120] -> w97
        tunnel: w81 -> [w118] mode=indexing
        n98 = Insert Menu Items(5:"Devices" ("menu tag"), 7:w118, 8:w118, 9:w121) -> (3:w120:refnum<k9>)  [unwired: 2 in, 2 out]
      }
      n99 = local write "fixsize"(w104) -> ()
      n100 = control-ref of="Pane 2"() -> (w100:refnum<vi>)
      n101 = property class="Pane"(reference=w100, "PaneColor"=u32 12369084) -> ()  [unwired: 1 in, 2 out]
      n102 = Enable Menu Tracking(4:w97) -> ()  [unwired: 2 in, 2 out]
      n103 = control-ref of="Channel"() -> (w86:refnum<vi>)
      n104 = control-ref of="This VI"() -> (w113:refnum<vi>)
      n105 = call "getNumberOFChannels.vi"("Device Name for vi mode"=w93) -> ("Number of channels"=w85:i32)  [unwired: 10 in]
      "Number of channels" <- w85
      n106 = call-poly <vilib>:"Ramp Pattern.vi"("start"=7 ("x"), "end"=w85, "delta"=1.0) -> ("Ramp Pattern"=w87:dbl[])  [unwired: 6 in, 2 out]
      n107 = property class="Ring (strict)"(reference=w89, "Disabled Items []"=w87) -> ()  [unwired: 1 in, 2 out]
      n108 = call "getPortAndIP.vi"("Device Name"=w93, "This Vi"=w113) -> ("Remote Host"=w95:string, "port or service name"=w94:u16, "reference out"=w111:refnum<vi>)  [unwired: 2 in, 2 out]
      "port or service name" <- w94
      "Remote Host" <- w95
      n109 = local read "showAll array"() -> (w92:refnum<vi>[])
      n110 = local read "enabled array"() -> (w91:refnum<vi>[])
      n111 = call "ConnectionFGV.vi"("command"=enum16{"get", "set", "init"}."set", "Remote Host in"=w95, "port or service name in"=w94) -> ()  [unwired: 7 in, 2 out]
      n112 = disable-structure shown="Disabled" {
        disable-tunnel: w115 -> [w127 _]
        disable-tunnel: w114 -> [w126 _]
        disable-tunnel: w111 -> [w124 _]
        frame Disabled {
          n113 = Unbundle By Name() -> ()  [unwired: 1 in, 2 out]
          n114 = control-ref of="Pane"() -> (w128:refnum<vi>)
          n115 = control-ref of="Pane 4"() -> (w125:refnum<vi>)
          n116 = call "reSizeSplitter.vi"("this vi"=w124, "pane"=w128, "left"=w127, "top"=w126, "Width"=u32 500, "Height"=u32 500, "pane2"=w125) -> ()  [unwired: 8 in, 1 out]
        }
        frame Enabled {
        }
      }
      n117 = property class="VI"(reference=w111, "Front Panel.Resizeable"=FALSE ("Front Panel Window:Resizable")) -> ()  [unwired: 1 in, 2 out]
      n118 = call "DiableEnumItems.vi"("Number Of Channels"=w85, "Enum in"=w86) -> ()  [unwired: 10 in]
      n119 = call "enableRefArray.vi"("Number of channels"=w85, "showAll array"=w91) -> ()  [unwired: 10 in]
      n120 = call "enableRefArray.vi"("Number of channels"=w85, "showAll array"=w92) -> ()  [unwired: 10 in]
      n121 = call "SetMultipleConnectionScope.vi"("Number of Connections size"=w85, "port or service name"=w94, "Remote Host"=w95) -> ()  [unwired: 9 in]
    }
    frame #1 {
      w146 = enum32{"All", "3Channels"}."All" ("NewVal")
      w164 = enum16{"get", "set", "init"}."init" ("Command")
      w170 = FALSE ("new Device Data")
      n122 = control-ref of="probeattenuation"() -> (w155:refnum<vi>)
      n123 = disable-structure shown="Disabled" {
        frame Disabled {
          n124 = control-ref of="This VI"() -> (w176:refnum<vi>)
          n125 = property class="VI"(reference=w176, "RT Menu Path"=path "C:/Users/loasis/Documents/000 LabView/Developers Version/Interface/GUI_Template/TemplateMenu.rtm" ("Run-Time Menu Path")) -> ()  [unwired: 1 in, 2 out]
        }
        frame Enabled {
        }
      }
      n126 = control-ref of="Impedance"() -> (w149:refnum<vi>)
      n127 = control-ref of="coupling"() -> (w152:refnum<vi>)
      n128 = control-ref of="offset"() -> (w151:refnum<vi>)
      n129 = control-ref of="channelenabled"() -> (w154:refnum<vi>)
      n130 = control-ref of="verticalrange"() -> (w153:refnum<vi>)
      n131 = local read "wavegaph array"() -> (w148:refnum<vi>[])
      n132 = control-ref of="All Channel"() -> (w147:refnum<vi>)
      n133 = local read "showAll array"() -> (w144:refnum<vi>[])
      n134 = Build Array(w152, w151, w153, w154, w155, w149) -> (→"indecator ref array":refnum<vi>[])
      n135 = local read "show3 array"() -> (w145:refnum<vi>[])
      n136 = call "setTraceVisib.vi"("showAll array 2"=w144, "show3 array 3"=w145, "NewVal"=w146, "All Channel"=w147, "wavegaph array 2"=w148) -> ()  [unwired: 7 in]
      n137 = local write "Display"(w146) -> ()
      n138 = call "ScopeTraceFGV.vi"("command"=enum16{"get", "set", "init"}."init", "Nr."=8) -> ()  [unwired: 8 in, 2 out]
      n139 = local write "image con closed 2"(w170) -> ()
      n140 = local write "image con closed"(w170) -> ()
      n141 = call "ClearBufferFGV.vi"("Command"=enum16{"set", "get", "init"}."init") -> ()  [unwired: 10 in, 1 out]
      n142 = local read "port or service name"() -> (w160:u16)
      n143 = call "WaitFGV.vi"("Command"=enum16{"get", "set", "init"}."set", "milliseconds to wait"="time to wait (TCP) 2") -> ()  [unwired: 9 in, 1 out]
      n144 = local write "shotnumber"(0 ("shotnumber")) -> ()
      n145 = call "ConnectionIDsFGV.vi"("Command"=enum16{"add", "get", "init"}."init") -> ()  [unwired: 10 in, 1 out]
      n146 = call "DATAStringFGV.vi"("Command"=enum16{"get", "set", "init"}."init") -> ()  [unwired: 9 in, 2 out]
      n147 = for {
        N: 8 -> [_]
        i -> [w173]
        n148 = call "multiple_ScopeTRace_FGV.vi"("Nr."=w173, "command"=commandForScopeTrace."init") -> ()  [unwired: 9 in, 1 out]
      }
      n149 = local write "Device Name (h)"("unknown" ("Device Name")) -> ()
      n150 = call "StatusImageConnectionFGV.vi"("Command"=w164) -> ()  [unwired: 10 in, 1 out]
      n151 = call "connectUDP.vi"("port or service name NOT USED"=w160) -> ("fast ID (h)"=w159:refnum<k16>, "slow ID (h)"=w158:refnum<k16>, "connections (hidden)"=→"connections (hidden)":variant[], "local Port"=→"local Port":u16)
      n152 = local write "Data String"("") -> ()
      n153 = call "StatusDataConnectionFGV.vi"("Command"=w164) -> ()  [unwired: 10 in, 1 out]
      n154 = call "StopFGV.vi"("Command"=enum16{"set", "get", "init"}."init") -> ()  [unwired: 9 in, 2 out]
      n155 = call "FastSlowFGV.vi"("Command"=enum16{"get", "set", "init"}."set", "slow ID"=w158, "fast ID"=w159) -> ()  [unwired: 7 in, 2 out]
      n156 = call "ScopeTraceConnectionArray_FGV.vi"("Command"=enum16{"add", "get", "init"}."init") -> ()  [unwired: 9 in, 2 out]
    }
    frame #2 {
      w215 = "Ch "  # Channel Selector
      n157 = local read "channelNames"() -> (w177:refnum<vi>[])
      n158 = local read "traces array"() -> (w197:refnum<vi>[])
      n159 = local read "indecator ref array"() -> (w211:refnum<vi>[])
      n160 = local read "horizontal ref"() -> (w210:refnum<vi>[])
      n161 = disable-structure shown="Disabled" {
        frame Disabled {
          n162 = local read "showAll array"() -> (w225:refnum<vi>[])
          n163 = call "createSubList_Scopes.vi"("showAll array"=w225) -> ()  [unwired: 10 in, 1 out]
        }
        frame Enabled {
        }
      }
      n164 = local read "enabled array"() -> (w200:refnum<vi>[])
      n165 = local read "Trigger ref"() -> (w209:refnum<vi>[])
      n166 = for {
        tunnel: w197 -> [w229] mode=indexing
        tunnel: "wait>>" -> [w228]
        tunnel: [w226] -> w195 mode=indexing
        n167 = property class="Clust (strict)"(reference=w229) -> ("Label.Text"=w227:string)  [unwired: 1 in, 2 out]
        n168 = Concatenate Strings(w228, w227) -> (w226:string)
      }
      n169 = Index Array(array=w195) -> (element #1=w194:string, element #2=w193:string, element #3=w192:string, element #4=w191:string, element #5=w190:string, element #6=w179:string, element #7=w189:string, element #8=w188:string)  [unwired: 8 in]
      n170 = Build Array (concatenate)(w177, w200, w210, w209) -> (w198:refnum<vi>[])
      n171 = local read "Trigger.Mode"() -> (w207:T10)
      n172 = local read "wavegaph array"() -> (w203:refnum<vi>[])
      n173 = Tick Count (ms)() -> (millisecond timer value=w220:u32)
      n174 = local read "showAll array"() -> (w178:refnum<vi>[])
      n175 = call "DataConnection_Multiple_Scope.vi"("Image Subscriber list"=w194, "showAll array"=w178, "Nr."=0) -> ()  [unwired: 9 in]
      n176 = call "DataConnection_Multiple_Scope.vi"("Image Subscriber list"=w193, "showAll array"=w178, "Nr."=1) -> ()  [unwired: 9 in]
      n177 = call "DataConnection_Multiple_Scope.vi"("Image Subscriber list"=w192, "showAll array"=w178, "Nr."=2) -> ()  [unwired: 9 in]
      n178 = call "DataConnection_Multiple_Scope.vi"("Image Subscriber list"=w191, "showAll array"=w178, "Nr."=3) -> ()  [unwired: 9 in]
      n179 = call "DataConnection_Multiple_Scope.vi"("Image Subscriber list"=w190, "showAll array"=w178, "Nr."=4) -> ()  [unwired: 9 in]
      n180 = call "DataConnection_Multiple_Scope.vi"("Image Subscriber list"=w179, "showAll array"=w178, "Nr."=5) -> ()  [unwired: 9 in]
      n181 = call "DataConnection_Multiple_Scope.vi"("Image Subscriber list"=w189, "showAll array"=w178, "Nr."=6) -> ()  [unwired: 9 in]
      n182 = call "DataConnection_Multiple_Scope.vi"("Image Subscriber list"=w188, "showAll array"=w178, "Nr."=7) -> ()  [unwired: 9 in]
      n183 = local read "enabled array"() -> (w204:refnum<vi>[])
      n184 = local read "show3 array"() -> (w202:refnum<vi>[])
      n185 = local read "traces array"() -> (w205:refnum<vi>[])
      n186 = local read "Trigger ref"() -> (w206:refnum<vi>[])
      n187 = call "getVarNamesGUI_WithSeperator.vi"("Channels"=string[] ["Channel1", "Channel0", "Channel2", "Channel3", "Channel4", "Channel5", "Channel6", "Channel7"], "Array"=w211) -> ("String"=w213:string)
      n188 = call "getVarNamesGUI.vi"("start"=FALSE, "Array"=w198) -> ("String"=w212:string)
      n189 = control-ref of="shotnumber"() -> (w218:refnum<vi>)
      n190 = control-ref of="Device Name (h)"() -> (w217:refnum<vi>)
      n191 = Concatenate Strings(w213, w212) -> (w199:string)
      "concatenated string" <- w199
      "basic sub." <- w199
      n192 = Build Array (concatenate)(w202, w178) -> (w201:refnum<vi>[])
      n193 = register-events(w211, w198, w201) -> (reference out=w216:refnum<event-registration>)  [unwired: 2 in, 1 out]
      n194 = call "setTriggerIndicatorVisible.vi"("NewVal"=w207, "Trigger ref"=w206) -> ()  [unwired: 10 in]
      n195 = call "DataConnection.vi"("Subscriber list"=w199, "Device Name (h)"=w217, "shotnumber"=w218) -> ()
      n196 = while {
        shift-right: [w255] -> w223
        shift-left: errorcluster {"status"=FALSE, "code"=0, "source"=""} ("error out") -> [_]
        tunnel: w211 -> [w265]
        shift-right: [w268] -> _
        shift-left: FALSE -> [w269]
        shift-right: [w267] -> _
        shift-left: w220 -> [w266]
        shift-right: [w260] -> _
        shift-left: "" ("Data String") -> [_]
        tunnel: w216 -> [w262]
        tunnel: w215 -> [_]
        tunnel: w198 -> [w254]
        shift-right: [w238] -> _
        shift-left: w207 -> [w249]
        tunnel: w206 -> [w248]
        tunnel: w205 -> [w237]
        tunnel: w204 -> [w236]
        tunnel: w178 -> [w230]
        tunnel: w202 -> [w233]
        tunnel: w203 -> [w232]
        stop <- w263 stop-if-true
        n197 = local read "Trigger.Mode"() -> (w247:T10)
        n198 = local read "Horizontal.Actual Sample Rate"() -> (w240:dbl)
        n199 = local read "Remote Host"() -> (w271:string)
        n200 = local read "Horizontal.Actual Record Length"() -> (w239:i32)
        n201 = Reciprocal(x=w240) -> (1/x=w242:dbl)
        "resolution" <- w242
        n202 = Multiply(x=w242, y=w239) -> (x*y=→"time wimdow":dbl)
        n203 = call "DATAStringFGV.vi"("Command"=enum16{"get", "set", "init"}."get") -> ("Data String out"=w252:string)  [unwired: 9 in, 1 out]
        "Data String" <- w252
        n204 = Not Equal?(x=w247, y=w249) -> (x != y?=w246:bool)
        n205 = First Call?() -> (First Call?: T/F=w231:bool)
        n206 = case shown="True" w231 {
          tunnel: w230 -> [_ w274]
          frame False {
          }
          frame True {
            n207 = call "GenEventDisplay.vi"("showAll array"=w274) -> ()  [unwired: 11 in]
          }
        }
        n208 = disable-structure shown="Disabled" {
          disable-tunnel: w237 -> [w292 _]
          disable-tunnel: w236 -> [w291 _]
          disable-tunnel: w230 -> [w290 _]
          disable-tunnel: [w287 _] -> w235
          disable-tunnel: [w286 _] -> w234
          frame Disabled {
            n209 = Equal?(y=enum32{"All", "3Channels"}."3Channels") -> (x = y?=w288:bool)  [unwired: 1 in]
            n210 = for {
              tunnel: w292 -> [w308] mode=indexing
              tunnel: w291 -> [w307] mode=indexing
              shift-right: [w305] -> w287
              shift-left: waveform(dbl)[] [] -> [w304]
              shift-right: [w302] -> w286
              shift-left: string[] [] -> [w301]
              tunnel: w290 -> [w300] mode=indexing
              tunnel: w288 -> [w296]
              n211 = property class="Bool (strict)"(reference=w300) -> ("Value"=w297:bool)  [unwired: 1 in, 2 out]
              n212 = property class="Bool (strict)"(reference=w307) -> ("Value"=w299:bool)  [unwired: 1 in, 2 out]
              n213 = property class="Clust (strict)"(reference=w308) -> ("Value"=w306:T2, "Label.Text"=w303:string)  [unwired: 1 in, 2 out]
              n214 = Or(x=w297, y=w296) -> (x .or. y?=w295:bool)
              n215 = And(x=w299, y=w295) -> (x .and. y?=w298:bool)
              n216 = case shown="True" w298 {
                tunnel: w306 -> [_ w319]
                tunnel: [w310 w317] -> w305
                tunnel: w304 -> [w310 w316]
                tunnel: w303 -> [_ w313]
                tunnel: [w309 w315] -> w302
                tunnel: w301 -> [w309 w314]
                frame False {
                }
                frame True {
                  n217 = Match Pattern(string=w313, regular expression="\\.") -> (after substring=w311:string)  [unwired: 1 in, 3 out]
                  n218 = call "ScopeWaveToTrace.vi"("scopeTrace.Channel0"=w319) -> ("Waveform"=w318:waveform(dbl))  [unwired: 10 in]
                  n219 = Build Array (concatenate)(w314, w311) -> (w315:string[])
                  n220 = Build Array (concatenate)(w316, w318) -> (w317:waveform(dbl)[])
                }
              }
            }
          }
          frame Enabled {
          }
        }
        n221 = call <userlib>:"Get Strings from Enum__ogtk.vi"("Enum"="Channel") -> ("String Value"=w253:string)  [unwired: 7 in, 3 out]
        n222 = event shown="[10] Menu Selection (User)" {
          selector: w262 -> [_ _ _ _ _ _ _ _ _ _ _]
          dyn-events: _ -> [_ _ _ _ _ _ _ _ _ _ _]
          timeout: "time to wait (main loop)" -> [_ _ _ _ _ _ _ _ _ _ _]
          tunnel: [_ _ _ _ w361 _ _ _ w424 w441 w499] -> w270
          tunnel: w271 -> [_ _ _ _ _ _ _ _ _ _ _]
          tunnel: "timeout ms (slow resp)" -> [_ _ _ _ _ _ _ _ _ _ _]
          tunnel: errorcluster {"status"=FALSE, "code"=0, "source"=""} ("error out") -> [_ _ _ _ w365 _ _ _ w426 w441 w500]
          tunnel: [_ _ _ _ TRUE _ _ _ TRUE _ _] -> w244
          tunnel: [_ _ _ _ _ _ _ _ _ _ w505] -> w263
          tunnel: [_ _ _ _ _ _ _ _ _ w440 w502] -> _
          tunnel: w269 -> [_ _ _ _ _ _ _ _ _ w440 _]
          tunnel: [TRUE _ _ _ _ _ _ _ _ _ _] -> w268
          tunnel: w253 -> [_ _ _ _ w363 _ _ _ _ _ _]
          tunnel: w230 -> [_ _ _ _ _ w377 _ _ _ w439 _]
          tunnel: w233 -> [_ _ _ _ _ w383 _ _ _ w438 _]
          tunnel: w232 -> [_ _ _ _ _ w384 _ _ _ _ _]
          event Panel Resize {
            n223 = event-data() -> ()  [unwired: 1 in, 7 out]
          }
          event "reset": Value Change {
            n224 = event-data() -> ()  [unwired: 1 in, 5 out]
            n225 = control-ref of="Channel"() -> (w331:refnum<vi>)
            n226 = local write "reset"(FALSE ("reset")) -> ()
            n227 = control-ref of="ChannelRing"() -> (w330:refnum<vi>)
            n228 = local read "showAll array"() -> (w334:refnum<vi>[])
            n229 = local read "port or service name"() -> (w336:u16)
            n230 = local read "Remote Host"() -> (w335:string)
            n231 = local read "enabled array"() -> (w332:refnum<vi>[])
            n232 = call "DiableEnumItems.vi"("Number Of Channels"=w327, "Enum in"=w331) -> ()  [unwired: 10 in]
            n233 = call "enableRefArray.vi"("Number of channels"=w327, "showAll array"=w332) -> ()  [unwired: 10 in]
            n234 = call "enableRefArray.vi"("Number of channels"=w327, "showAll array"=w334) -> ()  [unwired: 10 in]
            n235 = flat-sequence {
              tunnel: [w341] -> w327
              tunnel: [w341] -> w333
              tunnel: w336 -> [w346]
              tunnel: w335 -> [w347]
              tunnel: w333 -> [w345]
              frame #0 {
                n236 = local read "basic sub."() -> (w338:string)
                n237 = local read "showAll array"() -> (w339:refnum<vi>[])
                n238 = call "createSubList_Scopes.vi"("showAll array"=w339) -> ()  [unwired: 10 in, 1 out]
                n239 = call "SubScriberListGUI_FGV.vi"("Subscriber list"=w338, "Command"=enum16{"set", "get", "init"}."set") -> ()  [unwired: 9 in, 1 out]
              }
              frame #1 {
                n240 = local read "connections (hidden)"() -> (w344:variant[])
                n241 = control-ref of="Device Name (h)"() -> (w343:refnum<vi>)
                n242 = property class="Str"(reference=w343) -> ("Value"=w342:string)  [unwired: 1 in, 2 out]
                n243 = call "getNumberOFChannels.vi"("Device Name for vi mode"=w342) -> ("Number of channels"=w341:i32)  [unwired: 10 in]
                n244 = local write "Number of channels"(w341) -> ()
                n245 = call "Close UDP AND TCP connections.vi"("appended array"=w344) -> ()  [unwired: 7 in]
              }
              frame #2 {
                n246 = call "ConnectionFGV.vi"("command"=enum16{"get", "set", "init"}."set", "Remote Host in"=w347, "port or service name in"=w346) -> ("port or service name out"=w352:u16)  [unwired: 7 in, 1 out]
                n247 = call "SetMultipleConnectionScope.vi"("Number of Connections size"=w345, "port or service name"=w346, "Remote Host"=w347) -> ()  [unwired: 9 in]
                n248 = call "connectUDP.vi"("port or service name NOT USED"=w352) -> ("fast ID (h)"=w350:refnum<k16>, "slow ID (h)"=w349:refnum<k16>, "connections (hidden)"=w351:variant[])  [unwired: 1 out]
                n249 = local write "connections (hidden)"(w351) -> ()
                n250 = call "FastSlowFGV.vi"("Command"=enum16{"get", "set", "init"}."set", "slow ID"=w349, "fast ID"=w350) -> ()  [unwired: 7 in, 2 out]
              }
              frame #3 {
                n251 = Wait (ms)(milliseconds to wait=u32 500) -> ()  [unwired: 1 out]
              }
            }
            n252 = call-poly <vilib>:"Ramp Pattern.vi"("start"=w327, "end"=7 ("x"), "delta"=1.0) -> ("Ramp Pattern"=w326:dbl[])  [unwired: 6 in, 2 out]
            n253 = property class="Ring (strict)"(reference=w330, "Disabled Items []"=w326) -> ()  [unwired: 1 in, 2 out]
          }
          event "Display": Value Change {
            n254 = event-data() -> ("NewVal"=w358:enum32{"All", "3Channels"})  [unwired: 1 in, 4 out]
            n255 = local read "showAll array"() -> (w355:refnum<vi>[])
            n256 = local read "wavegaph array"() -> (w357:refnum<vi>[])
            n257 = local read "show3 array"() -> (w356:refnum<vi>[])
            n258 = control-ref of="All Channel"() -> (w359:refnum<vi>)
            n259 = call "setTraceVisib.vi"("showAll array 2"=w355, "show3 array 3"=w356, "NewVal"=w358, "All Channel"=w359, "wavegaph array 2"=w357) -> ()  [unwired: 7 in]
            n260 = call "GenEventDisplay.vi"("showAll array"=w355) -> ()  [unwired: 11 in]
          }
          event "Channel": Value Change {
            n261 = event-data() -> ("NewVal"=w360:T8)  [unwired: 1 in, 4 out]
            n262 = local write "ChannelRing"(w360) -> ()
          }
          event Value Change {
            n263 = event-data() -> ("CtlRef"=w369:refnum<vi>, "NewVal"=w368:variant)  [unwired: 1 in, 3 out]
            n264 = call "SendCommandEvent.vi"("error out 2"=w365, "Channel Selector"=w363, "NewVal"=w368, "CtlRef"=w369) -> ("error out"=w362:errorcluster, "error (h)"=→"error (h)":bool, "error message"=→"error message":string)  [unwired: 4 in, 1 out]
            n265 = flat-sequence {
              tunnel: w362 -> [w371]
              tunnel: [w371] -> w361
              frame #0 {
                n266 = Wait (ms)(milliseconds to wait=u32 200) -> ()  [unwired: 1 out]
              }
            }
          }
          event Value Change {
            n267 = event-data() -> ()  [unwired: 1 in, 5 out]
            n268 = local read "Display"() -> (w382:enum32{"All", "3Channels"})
            n269 = local read "channelNames"() -> (w376:refnum<vi>[])
            n270 = disable-structure shown="Disabled" {
              frame Disabled {
                n271 = control-ref of="reset"() -> (w417:refnum<vi>)
                n272 = property class="Bool (strict)"(reference=w417, "Val(Sgnl)"=TRUE ("Value (Signaling)")) -> ()  [unwired: 1 in, 2 out]
              }
              frame Enabled {
              }
            }
            n273 = Equal?(x=w382, y=enum32{"All", "3Channels"}."3Channels") -> (x = y?=w380:bool)
            n274 = case shown="False" w380 {
              tunnel: w384 -> [_ w403]
              tunnel: w383 -> [_ w402]
              tunnel: w377 -> [w396 w400]
              tunnel: [w396 w401] -> w378
              tunnel: w376 -> [w395 w398]
              frame False {
                n275 = control-ref of="All Channel"() -> (w397:refnum<vi>)
                n276 = call "NameAllGraph.vi"("channelNames 2"=w395, "showAll array"=w396, "WaveformGraph in"=w397) -> ()  [unwired: 9 in]
              }
              frame True {
                n277 = for {
                  tunnel: w400 -> [w406] mode=indexing
                  tunnel: [w404] -> w399 mode=indexing
                  n278 = property class="Bool (strict)"(reference=w406, "Value"=FALSE) -> (reference out=w404:refnum<vi>)  [unwired: 1 in, 1 out]
                }
                n279 = for {
                  tunnel: w402 -> [w415] mode=indexing
                  tunnel: w403 -> [w414] mode=indexing
                  tunnel: w399 -> [w411]
                  tunnel: [w411] -> w401
                  tunnel: w398 -> [w410]
                  n280 = property class="Enum (strict)"(reference=w415) -> ("Value"=w409:T8)  [unwired: 1 in, 2 out]
                  n281 = Index Array(array=w411, index=w409) -> (element=w413:refnum<vi>)
                  n282 = Index Array(array=w410, index=w409) -> (element=w408:refnum<vi>)
                  n283 = property class="Bool (strict)"(reference=w413, "Value"=TRUE) -> ()  [unwired: 1 in, 2 out]
                  n284 = property class="Str"(reference=w408) -> ("Value"=w407:string)  [unwired: 1 in, 2 out]
                  n285 = property class="WFGraph (strict)"(reference=w414, "Plot.Plot Name"=w407) -> ()  [unwired: 1 in, 2 out]
                }
              }
            }
            n286 = local read "channelNames"() -> (w375:refnum<vi>[])
            n287 = control-ref of="ChannelRing"() -> (w373:refnum<vi>)
            n288 = local read "Number of channels"() -> (w379:i32)
            n289 = for {
              tunnel: w375 -> [w386] mode=indexing
              tunnel: [w385] -> w374 mode=indexing
              n290 = property class="Str"(reference=w386) -> ("Value"=w385:string)  [unwired: 1 in, 2 out]
            }
            n291 = property class="Ring (strict)"(reference=w373, "Strings []"=w374) -> ("Value"=w372:u16)  [unwired: 1 in, 2 out]
            n292 = local write "Channel"(w372) -> ()
            n293 = for {
              N: w379 -> [_]
              tunnel: w378 -> [w388] mode=indexing
              i -> [w389]
              n294 = property class="Bool (strict)"(reference=w388) -> ("Value"=w387:bool)  [unwired: 1 in, 2 out]
              n295 = case shown="False" w387 {
                tunnel: w389 -> [w390 _]
                frame False {
                  n296 = call "ScopeTraceConnectionArray_FGV.vi"("Command"=enum16{"add", "get", "init"}."get", "Nr."=w390) -> ("connection ID out"=w391:refnum<k5>)  [unwired: 8 in, 1 out]
                  n297 = Not A Number/Path/Refnum?(number/path/refnum=w391) -> (NaN/Path/Refnum?=w392:bool)
                  n298 = case shown="False" w392 {
                    tunnel: w391 -> [w394 _]
                    frame False {
                      n299 = TCP Close Connection(connection ID=w394) -> ()  [unwired: 2 in, 2 out]
                    }
                    frame True {
                    }
                  }
                }
                frame True {
                }
              }
            }
          }
          event "ChannelRing": Value Change {
            n300 = event-data() -> ()  [unwired: 1 in, 5 out]
            n301 = local write "Channel"("ChannelRing") -> ()
          }
          event Value Change {
            n302 = event-data() -> ("NewVal"=w419:T10)  [unwired: 1 in, 4 out]
            n303 = disable-structure shown="Disabled" {
              disable-tunnel: w419 -> [w420 _]
              frame Disabled {
                n304 = local read "Trigger ref"() -> (w421:refnum<vi>[])
                n305 = call "setTriggerIndicatorVisible.vi"("NewVal"=w420, "Trigger ref"=w421) -> ()  [unwired: 10 in]
              }
              frame Enabled {
              }
            }
          }
          event Value Change {
            n306 = event-data() -> ("CtlRef"=w429:refnum<vi>, "NewVal"=w428:variant)  [unwired: 1 in, 3 out]
            n307 = call "SendCommandEvent.vi"("error out 2"=w426, "NewVal"=w428, "CtlRef"=w429) -> ("error out"=w425:errorcluster, "error (h)"=w422:bool, "error message"=w423:string)  [unwired: 5 in, 1 out]
            n308 = local write "error message"(w423) -> ()
            n309 = local write "error (h)"(w422) -> ()
            n310 = flat-sequence {
              tunnel: w425 -> [w431]
              tunnel: [w431] -> w424
              frame #0 {
                n311 = Wait (ms)(milliseconds to wait=u32 200) -> ()  [unwired: 1 out]
              }
            }
          }
          event Timeout {
            n312 = event-data() -> ()  [unwired: 1 in, 2 out]
            n313 = local read "Number of channels"() -> (w434:i32)
            n314 = Equal?(x="Display", y=enum32{"All", "3Channels"}."3Channels") -> (x = y?=w435:bool)
            n315 = case shown="False" w435 {
              tunnel: w439 -> [w447 _]
              tunnel: w438 -> [_ w480]
              tunnel: w434 -> [w445 w479]
              frame False {
                n316 = for {
                  N: w445 -> [_]
                  shift-right: [w454] -> w443
                  shift-left: waveform(dbl)[] [] -> [w455]
                  tunnel: w447 -> [w453] mode=indexing
                  tunnel: [TRUE] -> w444
                  i -> [w456]
                  n317 = property class="Bool (strict)"(reference=w453) -> ("Value"=w452:bool)  [unwired: 1 in, 2 out]
                  n318 = case shown="True" w452 {
                    tunnel: w456 -> [_ w465]
                    tunnel: w455 -> [w457 w461]
                    tunnel: [w457 w460] -> w454
                    frame False {
                    }
                    frame True {
                      n319 = call "multiple_ScopeTRace_FGV.vi"("Nr."=w465, "command"=commandForScopeTrace."get") -> ("output cluster 2"=w463:T21)  [unwired: 9 in]
                      n320 = Unbundle(w463) -> ("Info"=w462:T22, "Data"=w458:i16[])
                      n321 = Empty Array?(array=w458) -> (empty?=w459:bool)
                      n322 = case shown="False" w459 {
                        tunnel: w462 -> [w476 _]
                        tunnel: w461 -> [w475 w477]
                        tunnel: [w474 w477] -> w460
                        tunnel: w458 -> [w473 _]
                        frame False {
                          n323 = Unbundle By Name(w476) -> ("t0"=w467:dbl, "dt"=w472:dbl, "gain"=w469:dbl, "offset"=w470:dbl)  [unwired: 1 out]
                          n324 = To Time Stamp(1:w467) -> (0:w466:timestamp)
                          n325 = Bundle By Name("Y"=w473, "dt"=w472, "t0"=w466) -> (w471:waveform(i16))  [unwired: 1 in]
                          n326 = call <vilib>:"Waveform Scale and Offset.vi"("scale"=w469, "offset"=w470, "waveform in"=w471) -> ("waveform out"=w468:waveform(dbl))  [unwired: 7 in, 1 out]
                          n327 = Build Array (concatenate)(w475, w468) -> (w474:waveform(dbl)[])
                        }
                        frame True {
                        }
                      }
                    }
                  }
                }
                n328 = flat-sequence {
                  tunnel: w444 -> [_]
                  tunnel: w443 -> [w449]
                  tunnel: [w448] -> _
                  tunnel: w442 -> [w448]
                  frame #0 {
                  }
                  frame #1 {
                    n329 = case shown="False" w448 {
                      tunnel: w449 -> [w450 _]
                      frame False {
                        "All Channel" <- w450
                      }
                      frame True {
                      }
                    }
                  }
                }
                n330 = Empty Array?(array=w443) -> (empty?=w442:bool)
              }
              frame True {
                n331 = local read "wavegaph array"() -> (w478:refnum<vi>[])
                n332 = for {
                  N: w479 -> [_]
                  tunnel: w480 -> [w488] mode=indexing
                  tunnel: w478 -> [w481] mode=indexing
                  n333 = property class="Enum (strict)"(reference=w488) -> ("Value"=w482:T8)  [unwired: 1 in, 2 out]
                  n334 = call "multiple_ScopeTRace_FGV.vi"("Nr."=w482, "command"=commandForScopeTrace."get") -> ("output cluster 2"=w486:T21)  [unwired: 9 in]
                  n335 = Unbundle(w486) -> ("Info"=w485:T22, "Data"=w484:i16[])
                  n336 = Empty Array?(array=w484) -> (empty?=w483:bool)
                  n337 = case shown="False" w483 {
                    tunnel: w485 -> [w497 _]
                    tunnel: w484 -> [w495 _]
                    tunnel: w481 -> [w491 _]
                    frame False {
                      n338 = Unbundle By Name(w497) -> ("t0"=w489:dbl, "dt"=w496:dbl, "gain"=w493:dbl, "offset"=w494:dbl)  [unwired: 1 out]
                      n339 = Bundle By Name("dt"=w496, "Y"=w495) -> (w492:waveform(i16))  [unwired: 1 in]
                      n340 = call <vilib>:"Waveform Scale and Offset.vi"("scale"=w493, "offset"=w494, "waveform in"=w492) -> ("waveform out"=w490:waveform(dbl))  [unwired: 7 in, 1 out]
                      n341 = property class="WFGraph (strict)"(reference=w491, "Value"=w490, "XScale.Offset"=w489) -> ()  [unwired: 1 in, 2 out]
                    }
                    frame True {
                    }
                  }
                }
              }
            }
            n342 = call "StatusDataConnectionFGV.vi"("Command"=enum16{"get", "set", "init"}."get") -> ("Data Connection out"=→"Data Connection out":bool)  [unwired: 10 in]
          }
          event Menu Selection (User) {
            n343 = event-data() -> ("MenuRef"=w501:refnum<k9>, "ItemTag"=w503:string)  [unwired: 1 in, 3 out]
            n344 = control-ref of="Main Tap"() -> (w498:refnum<vi>)
            n345 = call "ChangeMainTap.vi"("error in"=w500, "ItemTag"=w503, "reference"=w498) -> ("error out"=w504:errorcluster, "Boolean"=w505:bool)
            n346 = case shown="Error" w504 {
              selector: w504 -> [w506 _]
              tunnel: w501 -> [_ w512]
              tunnel: [_ w514] -> w502
              tunnel: w503 -> [_ w513]
              tunnel: [w506 errorcluster {"status"=FALSE, "code"=0, "source"=""} ("error IO")] -> w499
              frame No Error {
              }
              frame Error {
                n347 = local read "All Devices (h)"() -> (w507:string[])
                n348 = call "disableMenueItem.vi"("ItemTag"=w513, "All Devices (h)"=w507, "MenuRef"=w512) -> ("this is a Device(tag)"=w511:bool, "menu reference out"=w510:refnum<k9>)  [unwired: 1 in, 1 out]
                n349 = Get Menu Item Info(7:w513, 11:w512) -> (2:w516:string, 4:w517:bool)  [unwired: 1 in, 5 out]
                n350 = Not(x=w517) -> (.not. x?=w515:bool)
                n351 = case shown="Default" w513 {
                  selector: w513 -> [_ w523 _ _ _ _]
                  tunnel: w515 -> [w518 w521 w533 _ _ _]
                  tunnel: [_ _ TRUE _ _ _] -> w514
                  tunnel: w511 -> [_ w524 _ _ _ _]
                  tunnel: [w518 w522 w533 _ _ _] -> w509
                  frame "fixsize" {
                    n352 = control-ref of="This VI"() -> (w520:refnum<vi>)
                    n353 = Not(x=w518) -> (.not. x?=w519:bool)
                    n354 = property class="VI"(reference=w520, "Front Panel.Resizeable"=w519) -> ()  [unwired: 1 in, 2 out]
                    "fixsize" <- w518
                  }
                  frame Default {
                    n355 = case shown="True" w524 {
                      tunnel: w523 -> [_ w525]
                      tunnel: [_ w527] -> w522
                      tunnel: w521 -> [_ w527]
                      frame False {
                      }
                      frame True {
                        n356 = control-ref of="reset"() -> (w529:refnum<vi>)
                        n357 = control-ref of="This VI"() -> (w532:refnum<vi>)
                        n358 = call "getPortAndIP.vi"("Device Name"=w525, "This Vi"=w532) -> ("Remote Host"=w531:string, "port or service name"=w530:u16)  [unwired: 2 in, 3 out]
                        n359 = local write "Device Name (h)"(w525) -> ()
                        n360 = local write "port or service name"(w530) -> ()
                        n361 = local write "Remote Host"(w531) -> ()
                        n362 = property class="Bool (strict)"(reference=w529, "Val(Sgnl)"=TRUE ("Value (Signaling)")) -> ()  [unwired: 1 in, 2 out]
                        n363 = Wait (ms)(milliseconds to wait=u32 100) -> ()  [unwired: 1 out]
                      }
                    }
                  }
                  frame "ratio" {
                    "ratio(h)" <- w533
                  }
                  frame "Local Saving Path" {
                    n364 = control-ref of="Local Saving Path"() -> (w535:refnum<vi>)
                    n365 = property class="Path"(reference=w535) -> (reference out=w538:refnum<vi>, "Value"=w539:path)  [unwired: 1 in, 1 out]
                    n366 = call "changePath.vi"("Local Saving in (h)"=w539) -> ("change (h)"=w537:bool, "Local Saving out (h)"=w536:path)  [unwired: 9 in]
                    n367 = case shown="True" w537 {
                      tunnel: w538 -> [_ w541]
                      tunnel: w536 -> [_ w540]
                      frame False {
                      }
                      frame True {
                        n368 = property class="Path"(reference=w541, "Val(Sgnl)"=w540) -> ()  [unwired: 1 in, 2 out]
                      }
                    }
                  }
                  frame "reset" {
                    n369 = control-ref of="reset"() -> (w543:refnum<vi>)
                    n370 = property class="Bool (strict)"(reference=w543, "Val(Sgnl)"=TRUE ("Value (Signaling)")) -> ()  [unwired: 1 in, 2 out]
                  }
                  frame "clear" {
                    n371 = control-ref of="reset"() -> (w545:refnum<vi>)
                    n372 = property class="Bool (strict)"(reference=w545, "Val(Sgnl)"=TRUE ("Value (Signaling)")) -> ()  [unwired: 1 in, 2 out]
                  }
                }
                n373 = Set Menu Item Info(6:w509, 7:w513, 10:w516, 11:w510) -> ()  [unwired: 3 in, 2 out]
              }
            }
          }
        }
        n374 = Not(x=w244) -> (.not. x?=w245:bool)
        n375 = And(x=w246, y=w245) -> (x .and. y?=w243:bool)
        n376 = case shown="True" w243 {
          tunnel: w248 -> [_ w322]
          tunnel: w247 -> [w320 w321]
          tunnel: [w320 w321] -> w238
          frame False {
          }
          frame True {
            n377 = call "setTriggerIndicatorVisible.vi"("NewVal"=w321, "Trigger ref"=w322) -> ()  [unwired: 10 in]
          }
        }
        n378 = control-ref of="error (h)"() -> (w258:refnum<vi>)
        n379 = control-ref of="error message"() -> (w259:refnum<vi>)
        n380 = disable-structure shown="Disabled" {
          disable-tunnel: w235 -> [_ _ _]
          disable-tunnel: w234 -> [w278 _ _]
          frame Disabled {
            n381 = control-ref of="All Channel"() -> (w277:refnum<vi>)
            n382 = for {
              tunnel: w278 -> [w281] mode=indexing
              tunnel: w277 -> [w280]
              tunnel: [w279] -> w276
              i -> [w279]
              n383 = property class="WFGraph (strict)"(reference=w280, "Active Plot"=w279, "Plot.Plot Name"=w281) -> ()  [unwired: 1 in, 2 out]
            }
            n384 = Increment(x=w276) -> (x+1=w275:i32)
            n385 = property class="WFGraph (strict)"(reference=w277, "LegNumRows"=w275) -> ()  [unwired: 1 in, 2 out]
            "Channel NAmes" <- w278
          }
          frame Disabled {
          }
          frame Enabled {
          }
        }
        n386 = call "updateInicatorsMainVi.vi"("Data String out"=w252, "Boolean"=w244, "Array"=w265, "Channel Selector"=w253, "error in"=w270) -> ("Data String out 2"=w260:string, "error out"=w256:errorcluster)  [unwired: 4 in, 1 out]
        n387 = call "error.vi"("Boolean"=w244, "millisecond timer value"=w266, "reference"=w258, "error message"=w259) -> ("millisecond timer value 2"=w267:u32)
        n388 = call "updateInicatorsMainVi.vi"("Data String out"=w252, "Boolean"=w244, "Array"=w254, "error in"=w256) -> ("name/data"=w251:string[][], "error out"=w255:errorcluster)  [unwired: 5 in, 1 out]
        "error out" <- w255
        n389 = case shown="False" "Y scale from range" {
          tunnel: w251 -> [_ w324]
          frame False {
          }
          frame True {
            n390 = local read "wavegaph array"() -> (w323:refnum<vi>[])
            n391 = call "setYrange.vi"("name/data"=w324, "Array"=w323) -> ()  [unwired: 9 in, 1 out]
          }
        }
        n392 = disable-structure shown="Disabled" {
          disable-tunnel: w235 -> [w285 _]
          disable-tunnel: w234 -> [w284 _]
          disable-tunnel: w233 -> [w283 _]
          disable-tunnel: w232 -> [w282 _]
          frame Disabled {
            n393 = call "assign3Graphs.vi"("wavegaph array in"=w282, "All Channel in 2"=w285, "channel name Array"=w284, "show3 array 2"=w283) -> ()  [unwired: 8 in]
          }
          frame Enabled {
          }
        }
        n394 = call "stop.vi"("Boolean"=w263) -> ()
      }
      n395 = local read "connections (hidden)"() -> (w222:variant[])
      n396 = call "Close UDP AND TCP connections.vi"("error in"=w223, "appended array"=w222) -> ()  [unwired: 6 in]
    }
    frame #3 {
      n397 = control-ref of="Main  Control"() -> (w547:refnum<vi>)
      n398 = property class="TabCtl (strict)"(reference=w547, "Tabs Visible?"=TRUE) -> ()  [unwired: 1 in, 2 out]
      n399 = property class="TabCtl (strict)"(reference=w547, "Tab Location"=enum32{"Top", "Bottom", "Left", "Right"}."Bottom") -> ()  [unwired: 1 in, 2 out]
      n400 = flat-sequence {
        frame #0 {
          n401 = Wait (ms)(milliseconds to wait=u32 0) -> ()  [unwired: 1 out]
        }
        frame #1 {
        }
        frame #2 {
          n402 = control-ref of="This VI"() -> (w553:refnum<vi>)
          n403 = case shown="True" FALSE {
            tunnel: w553 -> [w554 w557]
            tunnel: [w554 w555] -> w552
            frame False {
            }
            frame True {
              n404 = property class="VI" props=["Front Panel.Open"](reference=w557) -> (reference out=w556:refnum<vi>)  [unwired: 1 in, 2 out]
              n405 = invoke class="VI" method="FP.Close"(reference=w556) -> (reference out=w555:refnum<vi>)  [unwired: 2 in, 2 out]
            }
          }
          n406 = Close Reference(reference=w552) -> ()  [unwired: 1 in, 1 out]
          n407 = local write "All Channel"(waveform(dbl)[] [] ("All Channel")) -> ()
        }
      }
    }
  }
  n408 = control-ref of="show.1"() -> (w22:refnum<vi>)
  n409 = control-ref of="show.2"() -> (w21:refnum<vi>)
  n410 = Build Array(w22, w21) -> (→"show3 array":refnum<vi>[])
